vi "Athesim control.vi"() -> ()   [LabVIEW 2021]
uses:
  <vilib>/DAQmx/write.llb/DAQmx Write (Digital Bool 1Line 1Point).vi
  <vilib>/DAQmx/write.llb/DAQmx Write (Analog DBL 1Chan 1Samp).vi
  <vilib>/DAQmx/read.llb/DAQmx Read (Digital Bool 1Line 1Point).vi
  <vilib>/DAQmx/write.llb/DAQmx Write (Analog Wfm 1Chan NSamp).vi
  <vilib>/DAQmx/create/channels.llb/DAQmx Create Channel (DO-Digital Output).vi
  <vilib>/DAQmx/create/channels.llb/DAQmx Create Channel (DI-Digital Input).vi
  <vilib>/DAQmx/create/channels.llb/DAQmx Create Channel (AO-Voltage-Basic).vi
  <vilib>/DAQmx/miscellaneous.llb/DAQmx Fill In Error Info.vi
  <vilib>/Instr/_visa.llb/VISA Configure Serial Port (Instr).vi
  <vilib>/measure/NI_MABase.lvlib
panel:
  out "?":bool
  in  "Go live":bool
  in  "stop":bool=TRUE
  in  "Go SIM":bool
  in  "MG17Motor":refnum<k7>(container)
  in  "Tab Control":T1(tab)
  in  "Jog Z":bool
  in  "acquire 405":bool
  in  "405 Exp":dbl=150.0
  out "Images needed":dbl=216.0
  in  "5 phases":bool
  in  "Exposure time":dbl=100.0
  in  "interval /s":dbl
  in  "Timepoints":u32=8 min=1 max=1000 step=1
  in  "647":bool
  in  "561":bool
  in  "488":bool
  in  "405":bool
  in  "Steps /um":dbl
  in  "z-slices":dbl=1.0
  in  "acquire 640":bool
  in  "647 Exp":dbl=150.0
  in  "acquire 561":bool=TRUE
  in  "561 Exp":dbl=80.0
  in  "acquire 488":bool
  in  "488 Exp":dbl=40.0
  in  "Live mode":enum32{"Static", "Strobe", "Widefield", "SIM"}(radio)
  in  "Settle time":u32=60
  in  "Optosplit":T2(radio)=enum."rolling SIM"
  out "odd/even indicator":bool=TRUE
  out "Current voltage":dbl=0.95 format="%#_13g"
  in  "Boolean":bool
  in  "Radio Buttons":enum32{"V1", "V2", "V3"}(radio)
  in  "Debug":dbl[](array[numeric])=[0.95, 2.2, 3.45]
  in  "647 voltages":dbl[][](array[numeric])=[[0.95, 2.25, 3.5], [0.950655, 2.25185, 3.50055], [0.95131, 2.2537, 3.5011]]
  in  "561 voltages":dbl[][](array[numeric])=[[0.95, 2.2, 3.45], [0.9506, 2.2018, 3.451], [0.9512, 2.204, 3.452]]
  in  "488 voltages":dbl[][](array[numeric])=[[0.95, 2.25, 3.5], [0.951, 2.25185, 3.50055], [0.952, 2.2537, 3.5011]]
  in  "405 voltages":dbl[][](array[numeric])=[[1.0, 0.0, 0.0], [0.0, 0.0, 0.0], [0.0, 0.0, 4.0]]
  out "x+y":i32=5
  in  "647 voltages":dbl[][](array[numeric])=[[0.96, 2.2, 3.5], [0.97, 2.2035, 3.5085], [0.975, 2.2045, 3.5118]]
  in  "561 voltages":dbl[][](array[numeric])=[[0.85, 1.91, 3.2], [0.85065, 1.91064, 3.204], [0.85013, 1.91128, 3.208]]
  in  "488 voltages":dbl[][](array[numeric])=[[0.96, 2.2, 3.5], [0.97, 2.2045, 3.51], [0.975, 2.209, 3.52]]
  in  "405 voltages":dbl[][](array[numeric])=[[1.0, 0.0, 0.0], [0.0, 0.0, 0.0], [0.0, 0.0, 4.0]]
  in  "488 channel":refnum<visa-resource-name>="COM7"
  in  "488 power":dbl(slide)=5.627705627705628 min=0.0 max=100.0 step=0.05 scale=0.0..100.0
  in  "ASI stage channel":refnum<visa-resource-name>="COM3"
  in  "physical channels":tag="Dev1/ao0"
  in  "expose any":tag="Dev1/port0/line5"
  in  "647 Power":ext(slide)=31.05 scale=0.0..100.0
  in  "405 shutter":tag="Dev1/port0/line8"
  in  "561 shutter":tag="Dev1/port0/line0"
  in  "488 shutter":tag="Dev1/port0/line1"
  in  "Busy in":tag="Dev1/port0/line3"
  in  "Exposure out":tag="Dev1/port0/line2"
  in  "647 channel":refnum<visa-resource-name>="COM5"
  in  "561 power":dbl(slide)=31.16883116883117 min=0.0 max=100.0 step=0.05 scale=0.0..100.0
  in  "Tab Control 2":T3(tab)=enum."Page 5"
  out "Initialisation error":errorcluster
  out "stage error":errorcluster
  out "Camera/galvo error":errorcluster
  out "Laser error":errorcluster
  out "optosplit stage error":errorcluster
  out "resulting string":string="movrel z=0.000000 \r\n"
  out "resulting string 2":string="movrel z=-0.000000 \r\n"
  in  "short delay":dbl=5.0
  in  "long delay":dbl=55.0
  # "Acquire mode"
  # "o"
  # "o"
  # "o"
  # "o"
  # "o"
  # "o"
  # "o"
  # "o"
  # "o"
  # "o"
  # "o"
  # "o"
  # "-60"
  # "0"
  # "60"
  # "-60"
  # "0"
  # "60"
  # "-60"
  # "0"
  # "60"
  # "-60"
  # "0"
  # "60"
  # "0"
  # "2p/3"
  # "4p/3"
  # "o"
  # "o"
  # "o"
  # "o"
  # "o"
  # "o"
  # "o"
  # "o"
  # "o"
  # "o"
  # "o"
  # "o"
  # "-60"
  # "0"
  # "60"
  # "-60"
  # "0"
  # "60"
  # "-60"
  # "0"
  # "60"
  # "-60"
  # "0"
  # "60"
  # "0"
  # "3p/5"
  # "5p/5"
  # "7p/5"
  # "9p/5"
  # "Hardware lines"
  # "Laser control"
  # "Camera lines"
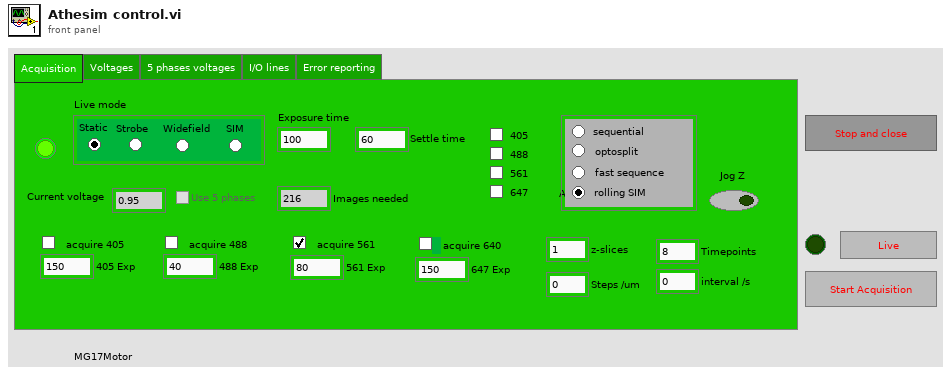
[diagram p1: front panel]
types:
  T1 = enum32{"Acquisition", "Voltages", "5 phases voltages", "I/O lines", "Error reporting"}
  T2 = enum32{"sequential", "optosplit", "fast sequence", "rolling SIM"}
  T3 = enum32{"Page 1", "Page 2", "Page 3", "Page 4", "Page 5"}
  T4 = enum8{"Enabled", "Disabled", "Disabled and Grayed Out"}
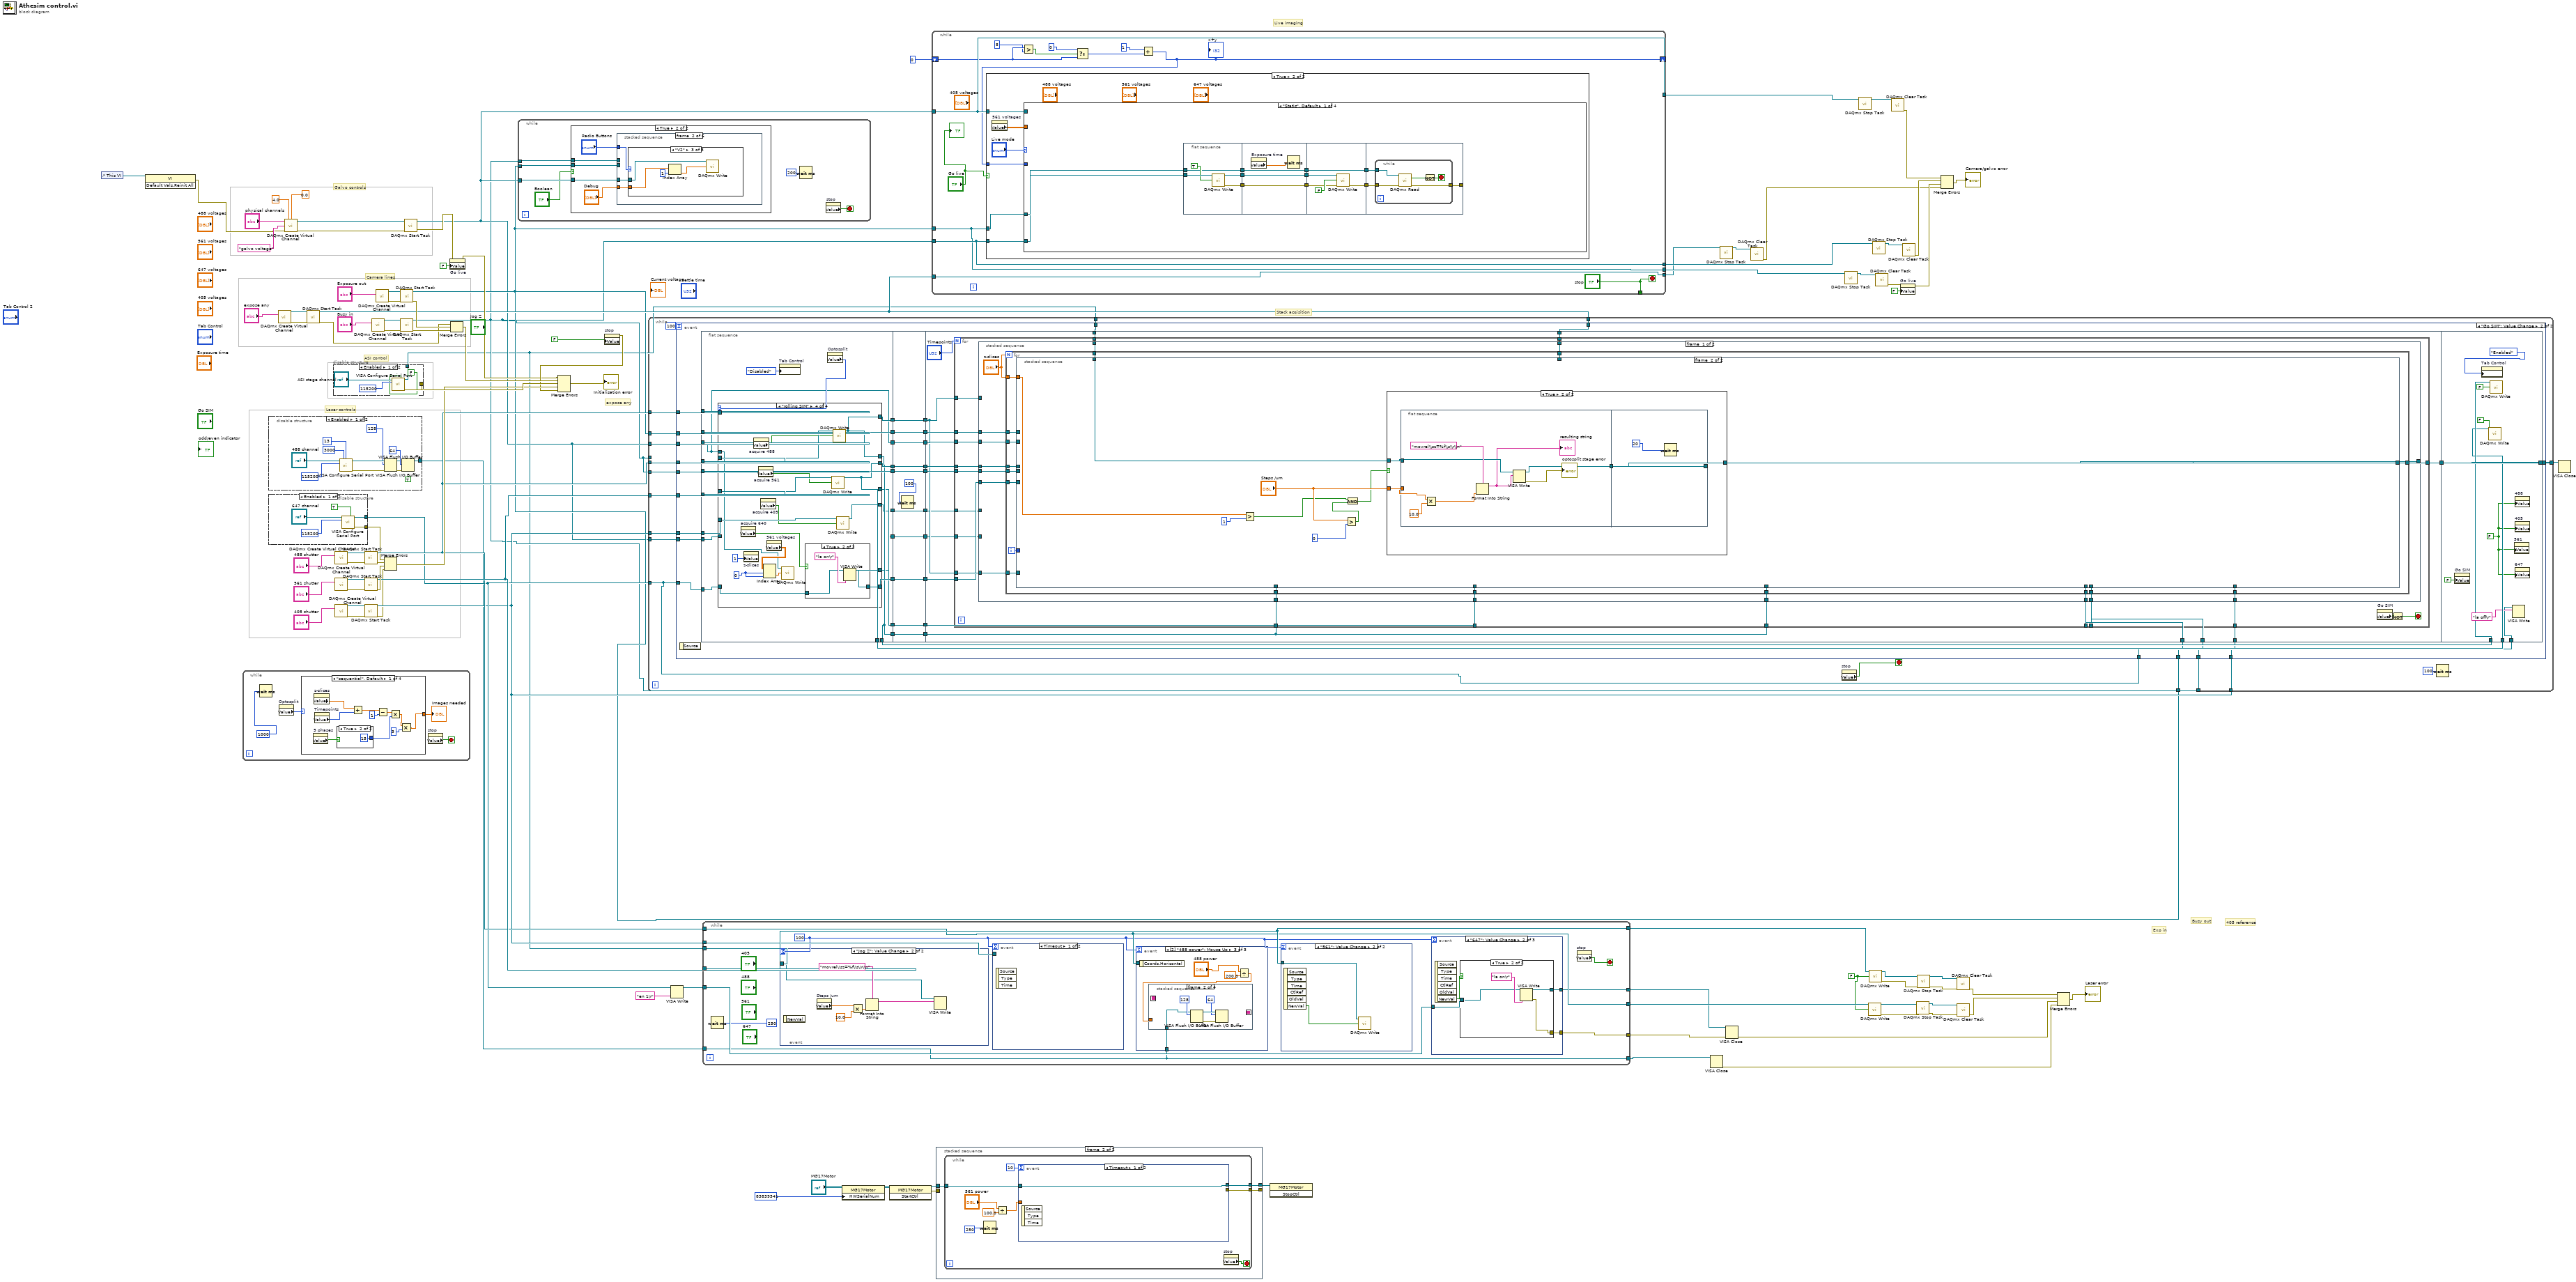
[diagram p0: block diagram]
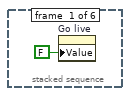
[diagram p4: hidden frame]
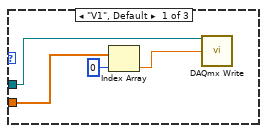
[diagram p5: hidden frame]
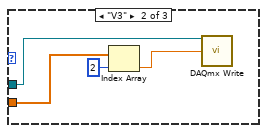
[diagram p6: hidden frame]
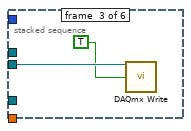
[diagram p7: hidden frame]
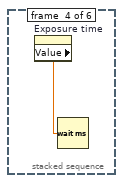
[diagram p8: hidden frame]
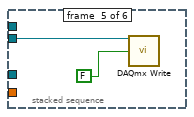
[diagram p9: hidden frame]
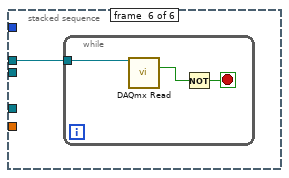
[diagram p10: hidden frame]
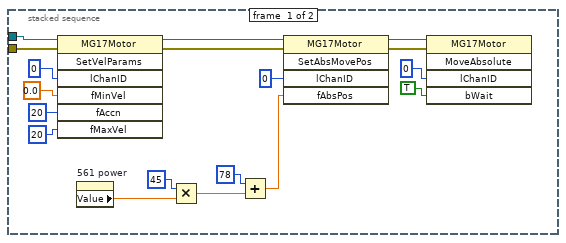
[diagram p11: hidden frame]
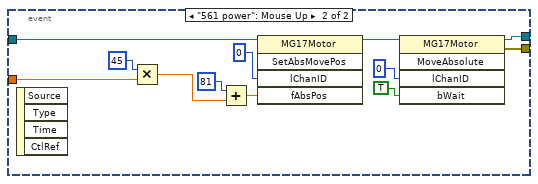
[diagram p12: hidden frame]
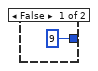
[diagram p14: hidden frame]
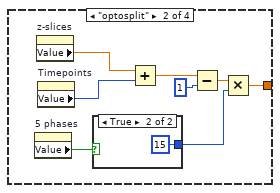
[diagram p15: hidden frame]
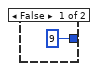
[diagram p16: hidden frame]
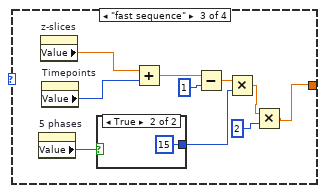
[diagram p17: hidden frame]
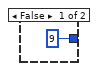
[diagram p18: hidden frame]
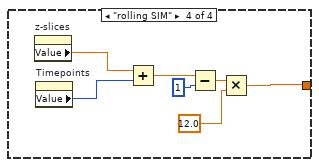
[diagram p19: hidden frame]
diagram:
  w63 = FALSE
  # "expose any"
  # "Busy out"
  # "Exp in"
  # "405 reference"
  # "Stack acqisition"
  # "Live imaging"
  # "Laser controls"
  # "ASI control"
  # "Camera lines"
  # "Galvo controls"
  n1 = control-ref of="This VI"() -> (w3:refnum<vi>)
  n2 = invoke class="VI" method="Default Vals.Reinit All"(reference=w3) -> (error out=w2:errorcluster)  [unwired: 2 in, 2 out]
  n3 = while {
    stop <- w99 stop-if-true
    n4 = Wait (ms)(milliseconds to wait=1000) -> ()  [unwired: 1 out]
    n5 = property on="Optosplit" class="RadioBtnsControl (strict)"() -> ("Value"=w98:T2)  [unwired: 2 in, 2 out]
    n6 = case shown="\"sequential\", Default" w98 {
      tunnel: [w101 w118 w123 w136] -> w100
      frame "sequential", Default {
        n7 = property on="5 phases" class="Bool (strict)"() -> ("Value"=w110:bool)  [unwired: 2 in, 2 out]
        n8 = property on="z-slices" class="DigNum (strict)"() -> ("Value"=w108:dbl)  [unwired: 2 in, 2 out]
        n9 = property on="Timepoints" class="DigNum (strict)"() -> ("Value"=w107:u32)  [unwired: 2 in, 2 out]
        n10 = case shown="True" w110 {
          tunnel: [9 15] -> w109
          frame False {
          }
          frame True {
          }
        }
        n11 = Add(x=w108, y=w107) -> (x+y=w105:dbl)
        n12 = Subtract(x=w105, y=1) -> (x-y=w104:dbl)
        n13 = Multiply(x=w104, y=w109) -> (x*y=w103:dbl)
        n14 = Multiply(x=w103, y=3) -> (x*y=w101:dbl)
      }
      frame "optosplit" {
        n15 = property on="5 phases" class="Bool (strict)"() -> ("Value"=w120:bool)  [unwired: 2 in, 2 out]
        n16 = property on="z-slices" class="DigNum (strict)"() -> ("Value"=w117:dbl)  [unwired: 2 in, 2 out]
        n17 = property on="Timepoints" class="DigNum (strict)"() -> ("Value"=w116:u32)  [unwired: 2 in, 2 out]
        n18 = case shown="True" w120 {
          tunnel: [9 15] -> w119
          frame False {
          }
          frame True {
          }
        }
        n19 = Add(x=w117, y=w116) -> (x+y=w114:dbl)
        n20 = Subtract(x=w114, y=1) -> (x-y=w113:dbl)
        n21 = Multiply(x=w113, y=w119) -> (x*y=w118:dbl)
      }
      frame "fast sequence" {
        n22 = property on="5 phases" class="Bool (strict)"() -> ("Value"=w132:bool)  [unwired: 2 in, 2 out]
        n23 = property on="z-slices" class="DigNum (strict)"() -> ("Value"=w130:dbl)  [unwired: 2 in, 2 out]
        n24 = property on="Timepoints" class="DigNum (strict)"() -> ("Value"=w129:u32)  [unwired: 2 in, 2 out]
        n25 = case shown="True" w132 {
          tunnel: [9 15] -> w131
          frame False {
          }
          frame True {
          }
        }
        n26 = Add(x=w130, y=w129) -> (x+y=w127:dbl)
        n27 = Subtract(x=w127, y=1) -> (x-y=w126:dbl)
        n28 = Multiply(x=w126, y=w131) -> (x*y=w125:dbl)
        n29 = Multiply(x=w125, y=2) -> (x*y=w123:dbl)
      }
      frame "rolling SIM" {
        n30 = property on="z-slices" class="DigNum (strict)"() -> ("Value"=w141:dbl)  [unwired: 2 in, 2 out]
        n31 = property on="Timepoints" class="DigNum (strict)"() -> ("Value"=w140:u32)  [unwired: 2 in, 2 out]
        n32 = Add(x=w141, y=w140) -> (x+y=w138:dbl)
        n33 = Subtract(x=w138, y=1) -> (x-y=w137:dbl)
        n34 = Multiply(x=w137, y=12.0) -> (x*y=w136:dbl)
      }
    }
    "Images needed" <- w100
    n35 = property on="stop" class="Bool (strict)"() -> ("Value"=w99:bool)  [unwired: 2 in, 2 out]
  }
  n36 = disable-structure shown="Enabled" {
    disable-tunnel: [w142 _] -> w7
    frame Enabled {
      (unwired) TRUE ("Enable Termination\nChar (T)")
      n37 = call-poly "VISA Configure Serial Port"("VISA resource name"="488 channel", "timeout (10sec)"=u32 3000, "termination char\n(0xA = '\\n' = LF)"=u8 13 ("termination char\n(0xA = '\\n' = LF)"), "baud rate (9600)"=u32 115200) -> ("VISA resource name out"=w152:refnum<visa-resource-name>, "error out"=w151:errorcluster)  [unwired: 5 in, 5 out]
      n38 = VISA Flush I/O Buffer(VISA resource name=w152, mask (16)=u16 128, error in (no error)=w151) -> (VISA resource name out=w148:refnum<visa-resource-name>, error out=w147:errorcluster)
      n39 = VISA Flush I/O Buffer(VISA resource name=w148, mask (16)=u16 64, error in (no error)=w147) -> (VISA resource name out=w142:refnum<visa-resource-name>)  [unwired: 1 out]
    }
    frame Disabled {
    }
  }
  n40 = disable-structure shown="Enabled" {
    disable-tunnel: [w154 _] -> w34
    disable-tunnel: [w153 _] -> w36
    frame Enabled {
      n41 = call-poly "VISA Configure Serial Port"("VISA resource name"="647 channel", "Enable Termination\nChar (T)"=TRUE ("Enable Termination\nChar (T)"), "baud rate (9600)"=u32 115200) -> ("VISA resource name out"=w154:refnum<visa-resource-name>, "error out"=w153:errorcluster)  [unwired: 11 in]
    }
    frame Disabled {
    }
  }
  n42 = call-poly <vilib>:"DAQmx Create Virtual Channel.vi"("lines"="expose any") -> ("task out"=w20:refnum<k21>, "error out"=w19:errorcluster)  [unwired: 13 in]
  n43 = call-poly <vilib>:"DAQmx Create Virtual Channel.vi"("maximum value"=4.0, "minimum value"=0.0, "physical channels"="physical channels", "name to assign"="galvo voltage", "error in"=w2) -> ("task out"=w13:refnum<k21>, "error out"=w12:errorcluster)  [unwired: 9 in]
  n44 = call <vilib>:"DAQmx Start Task.vi"("task/channels in"=w20, "error in"=w19) -> ("task out"=w17:refnum<k21>, "error out"=w18:errorcluster)  [unwired: 12 in]
  n45 = disable-structure shown="Enabled" {
    disable-tunnel: [w160 _] -> w80
    disable-tunnel: [w159 _] -> w1
    frame Enabled {
      n46 = call-poly "VISA Configure Serial Port"("VISA resource name"="ASI stage channel", "Enable Termination\nChar (T)"=FALSE, "baud rate (9600)"=u32 115200) -> ("VISA resource name out"=w159:refnum<visa-resource-name>, "error out"=w160:errorcluster)  [unwired: 11 in]
    }
    frame Disabled {
    }
  }
  n47 = call-poly <vilib>:"DAQmx Create Virtual Channel.vi"("lines"="488 shutter") -> ("task out"=w91:refnum<k21>, "error out"=w92:errorcluster)  [unwired: 13 in]
  n48 = call-poly <vilib>:"DAQmx Create Virtual Channel.vi"("lines"="561 shutter") -> ("task out"=w89:refnum<k21>, "error out"=w90:errorcluster)  [unwired: 13 in]
  n49 = call-poly <vilib>:"DAQmx Create Virtual Channel.vi"("lines"="405 shutter") -> ("task out"=w46:refnum<k21>, "error out"=w47:errorcluster)  [unwired: 13 in]
  n50 = call <vilib>:"DAQmx Start Task.vi"("task/channels in"=w91, "error in"=w92) -> ("task out"=w75:refnum<k21>, "error out"=w84:errorcluster)  [unwired: 12 in]
  n51 = call <vilib>:"DAQmx Start Task.vi"("task/channels in"=w89, "error in"=w90) -> ("task out"=w76:refnum<k21>, "error out"=w83:errorcluster)  [unwired: 12 in]
  n52 = call <vilib>:"DAQmx Start Task.vi"("task/channels in"=w46, "error in"=w47) -> ("task out"=w32:refnum<k21>, "error out"=w8:errorcluster)  [unwired: 12 in]
  n53 = call-poly <vilib>:"DAQmx Create Virtual Channel.vi"("lines"="Busy in") -> ("task out"=w93:refnum<k21>, "error out"=w94:errorcluster)  [unwired: 13 in]
  n54 = call-poly <vilib>:"DAQmx Create Virtual Channel.vi"("lines"="Exposure out") -> ("task out"=w96:refnum<k21>, "error out"=w95:errorcluster)  [unwired: 13 in]
  n55 = Merge Errors(w36, w84, w83, w8) -> (w78:errorcluster)
  n56 = call <vilib>:"DAQmx Start Task.vi"("task/channels in"=w96, "error in"=w95) -> ("task out"=w10:refnum<k21>, "error out"=w82:errorcluster)  [unwired: 12 in]
  n57 = call <vilib>:"DAQmx Start Task.vi"("task/channels in"=w93, "error in"=w94) -> ("task out"=w4:refnum<k21>, "error out"=w81:errorcluster)  [unwired: 12 in]
  n58 = call <vilib>:"DAQmx Start Task.vi"("task/channels in"=w13, "error in"=w12) -> ("task out"=w9:refnum<k21>, "error out"=w30:errorcluster)  [unwired: 12 in]
  n59 = property on="Go live" class="Bool (strict)"(error in=w30, "Value"=FALSE) -> (error out=w29:errorcluster)  [unwired: 1 in, 1 out]
  n60 = Merge Errors(w18, w82, w81) -> (w79:errorcluster)
  n61 = while {
    tunnel: w10 -> [w167]
    tunnel: w4 -> [w166]
    tunnel: w9 -> [w165]
    stop <- w168 stop-if-true
    n62 = case shown="True" "Boolean" {
      tunnel: w167 -> [_ w173]
      tunnel: w166 -> [_ w172]
      tunnel: w165 -> [_ w171]
      frame False {
      }
      frame True {
        n63 = stacked-sequence {
          tunnel: w173 -> [_ _ w191 _ w193 _]
          tunnel: w172 -> [_ _ _ _ _ w195]
          tunnel: "Radio Buttons" -> [_ w177 _ _ _ _]
          tunnel: "Debug" -> [_ w176 _ _ _ _]
          tunnel: w171 -> [_ w175 _ _ _ _]
          frame #0 {
            n64 = property on="Go live" class="Bool (strict)"("Value"=FALSE ("Go live")) -> ()  [unwired: 2 in, 2 out]
          }
          frame #1 {
            n65 = case shown="\"V2\"" w177 {
              tunnel: w176 -> [w180 w184 w188]
              tunnel: w175 -> [w181 w185 w189]
              frame "V1", Default {
                n66 = Index Array(array=w180, index=0) -> (element=w179:dbl)
                n67 = call-poly <vilib>:"DAQmx Write.vi"("task/channels in"=w181, "data"=w179) -> ()  [unwired: 11 in, 3 out]
              }
              frame "V3" {
                n68 = Index Array(array=w184, index=2) -> (element=w183:dbl)
                n69 = call-poly <vilib>:"DAQmx Write.vi"("task/channels in"=w185, "data"=w183) -> ()  [unwired: 11 in, 3 out]
              }
              frame "V2" {
                n70 = Index Array(array=w188, index=1) -> (element=w187:dbl)
                n71 = call-poly <vilib>:"DAQmx Write.vi"("task/channels in"=w189, "data"=w187) -> ()  [unwired: 11 in, 3 out]
              }
            }
          }
          frame #2 {
            n72 = call-poly <vilib>:"DAQmx Write.vi"("task/channels in"=w191, "data"=TRUE) -> ()  [unwired: 11 in, 3 out]
          }
          frame #3 {
            n73 = property on="Exposure time" class="DigNum (strict)"() -> ("Value"=w192:dbl)  [unwired: 2 in, 2 out]
            n74 = Wait (ms)(milliseconds to wait=w192) -> ()  [unwired: 1 out]
          }
          frame #4 {
            n75 = call-poly <vilib>:"DAQmx Write.vi"("task/channels in"=w193, "data"=FALSE) -> ()  [unwired: 11 in, 3 out]
          }
          frame #5 {
            n76 = while {
              tunnel: w195 -> [w196]
              stop <- w198 stop-if-true
              n77 = call-poly <vilib>:"DAQmx Read.vi"("task/channels in"=w196) -> ("data"=w197:bool)  [unwired: 12 in, 2 out]
              n78 = Not(x=w197) -> (.not. x?=w198:bool)
            }
          }
        }
      }
    }
    n79 = Wait (ms)(milliseconds to wait=u32 200) -> ()  [unwired: 1 out]
    n80 = property on="stop" class="Bool (strict)"() -> ("Value"=w168:bool)  [unwired: 2 in, 2 out]
  }
  n81 = property on="stop" class="Bool (strict)"("Value"=FALSE) -> (error out=w49:errorcluster)  [unwired: 2 in, 1 out]
  n82 = Merge Errors(w29, w79, w80, w78, w49) -> (→"Initialisation error":errorcluster)
  n83 = while {
    tunnel: w10 -> [w215]
    tunnel: w4 -> [w214]
    tunnel: w9 -> [w213]
    tunnel: w75 -> [w212]
    tunnel: w76 -> [w211]
    tunnel: w75 -> [w210]
    tunnel: w1 -> [w208]
    tunnel: [w207] -> w51
    tunnel: w4 -> [_]
    tunnel: w34 -> [w205]
    tunnel: w32 -> [w206]
    tunnel: w32 -> [w204]
    tunnel: w10 -> [w203]
    tunnel: w4 -> [w202]
    tunnel: w9 -> [w201]
    tunnel: w17 -> [w200]
    stop <- w209 stop-if-true
    n84 = event shown="[1] \"Go SIM\": Value Change" {
      selector: _ -> [_ _]
      dyn-events: _ -> [_ _]
      timeout: 100 -> [_ _]
      tunnel: w215 -> [_ w256]
      tunnel: w214 -> [_ w255]
      tunnel: w213 -> [_ w254]
      tunnel: w212 -> [_ w253]
      tunnel: w211 -> [_ w252]
      tunnel: w210 -> [_ w251]
      tunnel: w208 -> [w217 w250]
      tunnel: [w217 w249] -> w207
      tunnel: w205 -> [_ w245]
      tunnel: w206 -> [_ w244]
      tunnel: w205 -> [_ w243]
      tunnel: w204 -> [_ w242]
      tunnel: w203 -> [_ w241]
      tunnel: w202 -> [_ w240]
      tunnel: w201 -> [_ w239]
      tunnel: w200 -> [_ w218]
      event Timeout {
        n85 = event-data() -> ()  [unwired: 1 in, 3 out]
      }
      event "Go SIM": Value Change {
        n86 = event-data() -> ()  [unwired: 1 in, 1 out]
        n87 = flat-sequence {
          tunnel: [w274] -> w238
          tunnel: w256 -> [w274]
          tunnel: [w273] -> w236
          tunnel: w255 -> [w273]
          tunnel: [w258] -> w234
          tunnel: w254 -> [w258]
          tunnel: w253 -> [w271]
          tunnel: w252 -> [w270]
          tunnel: w251 -> [w269]
          tunnel: [w268] -> w232
          tunnel: [w267] -> w230
          tunnel: [w263] -> w246
          tunnel: [w262] -> w247
          tunnel: w245 -> [w266]
          tunnel: w244 -> [w265]
          tunnel: [w264] -> w228
          tunnel: [w263] -> w226
          tunnel: [w262] -> w224
          tunnel: w239 -> [w261]
          tunnel: [w260] -> w221
          tunnel: [w259] -> w219
          tunnel: w238 -> [w364]
          tunnel: [w364] -> w237
          tunnel: w236 -> [w363]
          tunnel: [w363] -> w235
          tunnel: w234 -> [w362]
          tunnel: [w362] -> w233
          tunnel: w232 -> [w361]
          tunnel: [w361] -> w231
          tunnel: w230 -> [w360]
          tunnel: [w360] -> w229
          tunnel: w228 -> [w359]
          tunnel: [w359] -> w227
          tunnel: w226 -> [w358]
          tunnel: [w358] -> w225
          tunnel: w224 -> [w357]
          tunnel: [w357] -> w223
          tunnel: [w355] -> w222
          tunnel: w221 -> [w355]
          tunnel: [w354] -> w220
          tunnel: w219 -> [w354]
          tunnel: w237 -> [w381]
          tunnel: w235 -> [w380]
          tunnel: w233 -> [w379]
          tunnel: w231 -> [w378]
          tunnel: w229 -> [w369]
          tunnel: w250 -> [w377]
          tunnel: [w376] -> w248
          tunnel: w227 -> [w375]
          tunnel: w225 -> [w373]
          tunnel: w223 -> [w374]
          tunnel: w242 -> [w372]
          tunnel: w241 -> [w371]
          tunnel: w240 -> [w370]
          tunnel: w222 -> [w368]
          tunnel: w220 -> [w367]
          tunnel: w218 -> [w366]
          tunnel: [w1177] -> w249
          tunnel: w248 -> [w1177]
          tunnel: w247 -> [w1173]
          tunnel: w246 -> [w1174]
          tunnel: w243 -> [w1171]
          frame #0 {
            n88 = property on="Tab Control" class="TabCtl (strict)"("DisabledEnum"=T4."Disabled" ("Disabled")) -> ()  [unwired: 2 in, 2 out]
            n89 = property on="Optosplit" class="RadioBtnsControl (strict)"() -> ("Value"=w272:T2)  [unwired: 2 in, 2 out]
            n90 = case shown="\"rolling SIM\"" w272 {
              tunnel: w271 -> [_ _ _ _]
              tunnel: w270 -> [w285 w307 w326 w345]
              tunnel: w269 -> [w286 w308 w328 w347]
              tunnel: [w284 w306 w325 w344] -> w268
              tunnel: [w283 w305 w327 w346] -> w267
              tunnel: [w284 w306 w325 w344] -> w262
              tunnel: [w283 w305 w327 w346] -> w263
              tunnel: w266 -> [w278 w300 w323 w343]
              tunnel: w265 -> [w281 w303 w321 w342]
              tunnel: [w275 w297 w319 w340] -> w264
              tunnel: [w279 w301 w320 w341] -> w260
              tunnel: w261 -> [w276 w299 _ _]
              tunnel: [w275 w297 w319 w340] -> w259
              tunnel: w258 -> [_ _ _ w331]
              frame "sequential", Default {
                n91 = property on="odd/even indicator" class="Bool (strict)"() -> ("Value"=w277:bool)  [unwired: 2 in, 2 out]
                n92 = case shown="True" w277 {
                  tunnel: w276 -> [w292 w296]
                  frame False {
                    w290 = 2
                    n93 = property on="647 voltages" class="Arr (strict)"() -> ("Value"=w291:dbl[][])  [unwired: 2 in, 2 out]
                    n94 = Index Array(array=w291, index (row)=w290, index (col)=w290) -> (element=w289:dbl)
                    n95 = call-poly <vilib>:"DAQmx Write.vi"("task/channels in"=w292, "data"=w289) -> ()  [unwired: 11 in, 3 out]
                  }
                  frame True {
                    w294 = 0
                    n96 = property on="561 voltages" class="Arr (strict)"() -> ("Value"=w295:dbl[][])  [unwired: 2 in, 2 out]
                    n97 = Index Array(array=w295, index (row)=w294, index (col)=w294) -> (element=w293:dbl)
                    n98 = call-poly <vilib>:"DAQmx Write.vi"("task/channels in"=w296, "data"=w293) -> ()  [unwired: 11 in, 3 out]
                  }
                }
                n99 = call-poly <vilib>:"DAQmx Write.vi"("task/channels in"=w281, "data"=FALSE) -> ("task out"=w279:refnum<k21>)  [unwired: 11 in, 2 out]
                n100 = call-poly <vilib>:"DAQmx Write.vi"("task/channels in"=w285, "data"=FALSE) -> ("task out"=w284:refnum<k21>)  [unwired: 11 in, 2 out]
                n101 = call-poly <vilib>:"DAQmx Write.vi"("task/channels in"=w286, "data"=FALSE) -> ("task out"=w283:refnum<k21>)  [unwired: 11 in, 2 out]
                n102 = VISA Write(VISA resource name=w278, write buffer="la off\r" ("format string")) -> (VISA resource name out=w275:refnum<visa-resource-name>)  [unwired: 1 in, 2 out]
              }
              frame "fast sequence" {
                n103 = property on="odd/even indicator" class="Bool (strict)"() -> ("Value"=w298:bool)  [unwired: 2 in, 2 out]
                n104 = case shown="True" w298 {
                  tunnel: w299 -> [w314 w318]
                  frame False {
                    w312 = 2
                    n105 = property on="647 voltages" class="Arr (strict)"() -> ("Value"=w313:dbl[][])  [unwired: 2 in, 2 out]
                    n106 = Index Array(array=w313, index (row)=w312, index (col)=w312) -> (element=w311:dbl)
                    n107 = call-poly <vilib>:"DAQmx Write.vi"("task/channels in"=w314, "data"=w311) -> ()  [unwired: 11 in, 3 out]
                  }
                  frame True {
                    w316 = 0
                    n108 = property on="647 voltages" class="Arr (strict)"() -> ("Value"=w317:dbl[][])  [unwired: 2 in, 2 out]
                    n109 = Index Array(array=w317, index (row)=w316, index (col)=w316) -> (element=w315:dbl)
                    n110 = call-poly <vilib>:"DAQmx Write.vi"("task/channels in"=w318, "data"=w315) -> ()  [unwired: 11 in, 3 out]
                  }
                }
                n111 = call-poly <vilib>:"DAQmx Write.vi"("task/channels in"=w303, "data"=FALSE) -> ("task out"=w301:refnum<k21>)  [unwired: 11 in, 2 out]
                n112 = call-poly <vilib>:"DAQmx Write.vi"("task/channels in"=w307, "data"=FALSE) -> ("task out"=w306:refnum<k21>)  [unwired: 11 in, 2 out]
                n113 = call-poly <vilib>:"DAQmx Write.vi"("task/channels in"=w308, "data"=FALSE) -> ("task out"=w305:refnum<k21>)  [unwired: 11 in, 2 out]
                n114 = VISA Write(VISA resource name=w300, write buffer="la off\r" ("format string")) -> (VISA resource name out=w297:refnum<visa-resource-name>)  [unwired: 1 in, 2 out]
              }
              frame "optosplit" {
                n115 = call-poly <vilib>:"DAQmx Write.vi"("task/channels in"=w326, "data"=TRUE) -> ("task out"=w325:refnum<k21>)  [unwired: 11 in, 2 out]
                n116 = call-poly <vilib>:"DAQmx Write.vi"("task/channels in"=w328, "data"=TRUE) -> ("task out"=w327:refnum<k21>)  [unwired: 11 in, 2 out]
                n117 = call-poly <vilib>:"DAQmx Write.vi"("task/channels in"=w321, "data"=TRUE) -> ("task out"=w320:refnum<k21>)  [unwired: 11 in, 2 out]
                n118 = VISA Write(VISA resource name=w323, write buffer="la on\r" ("format string")) -> (VISA resource name out=w319:refnum<visa-resource-name>)  [unwired: 1 in, 2 out]
              }
              frame "rolling SIM" {
                w336 = 0
                n119 = property on="acquire 640" class="Bool (strict)"() -> ("Value"=w332:bool)  [unwired: 2 in, 2 out]
                n120 = property on="z-slices" class="DigNum (strict)"("Value"=1) -> ()  [unwired: 2 in, 2 out]
                n121 = property on="acquire 488" class="Bool (strict)"() -> ("Value"=w335:bool)  [unwired: 2 in, 2 out]
                n122 = property on="acquire 561" class="Bool (strict)"() -> ("Value"=w334:bool)  [unwired: 2 in, 2 out]
                n123 = property on="acquire 405" class="Bool (strict)"() -> ("Value"=w333:bool)  [unwired: 2 in, 2 out]
                n124 = property on="561 voltages" class="Arr (strict)"() -> ("Value"=w337:dbl[][])  [unwired: 2 in, 2 out]
                n125 = Index Array(array=w337, index (row)=w336, index (col)=w336) -> (element=w338:dbl)
                n126 = call-poly <vilib>:"DAQmx Write.vi"("task/channels in"=w331, "data"=w338) -> ()  [unwired: 11 in, 3 out]
                n127 = case shown="True" w332 {
                  tunnel: w343 -> [w349 w352]
                  tunnel: [w348 w351] -> w340
                  frame False {
                    n128 = VISA Write(VISA resource name=w349, write buffer="la off\r" ("format string")) -> (VISA resource name out=w348:refnum<visa-resource-name>)  [unwired: 1 in, 2 out]
                  }
                  frame True {
                    n129 = VISA Write(VISA resource name=w352, write buffer="la on\r" ("format string")) -> (VISA resource name out=w351:refnum<visa-resource-name>)  [unwired: 1 in, 2 out]
                  }
                }
                n130 = call-poly <vilib>:"DAQmx Write.vi"("task/channels in"=w345, "data"=w334) -> ("task out"=w344:refnum<k21>)  [unwired: 11 in, 2 out]
                n131 = call-poly <vilib>:"DAQmx Write.vi"("task/channels in"=w347, "data"=w335) -> ("task out"=w346:refnum<k21>)  [unwired: 11 in, 2 out]
                n132 = call-poly <vilib>:"DAQmx Write.vi"("task/channels in"=w342, "data"=w333) -> ("task out"=w341:refnum<k21>)  [unwired: 11 in, 2 out]
              }
            }
          }
          frame #1 {
            n133 = Wait (ms)(milliseconds to wait=100) -> ()  [unwired: 1 out]
          }
          frame #2 {
            n134 = for {
              N: "Timepoints" -> [_]
              tunnel: w381 -> [w401]
              tunnel: w380 -> [w400]
              tunnel: w379 -> [w399]
              tunnel: w378 -> [w398]
              tunnel: w369 -> [w397]
              tunnel: w377 -> [w396]
              tunnel: [w395] -> w376
              tunnel: w375 -> [w394]
              tunnel: w374 -> [w393]
              tunnel: w373 -> [w392]
              tunnel: w373 -> [w391]
              tunnel: w372 -> [w390]
              tunnel: w371 -> [w389]
              tunnel: w370 -> [w388]
              tunnel: w369 -> [w387]
              tunnel: w368 -> [w386]
              tunnel: w367 -> [w385]
              tunnel: w366 -> [w384]
              stop <- w382 stop-if-true
              n135 = stacked-sequence {
                tunnel: w401 -> [w417 _]
                tunnel: w400 -> [w416 _]
                tunnel: w399 -> [w415 _]
                tunnel: w398 -> [w414 w1081]
                tunnel: w397 -> [w413 _]
                tunnel: w396 -> [w412 w1083]
                tunnel: [w411 _] -> w395
                tunnel: w394 -> [w410 _]
                tunnel: w393 -> [w409 _]
                tunnel: w392 -> [w408 _]
                tunnel: w391 -> [w407 _]
                tunnel: w390 -> [w406 _]
                tunnel: w389 -> [w405 _]
                tunnel: w388 -> [w404 _]
                tunnel: w387 -> [_ w1082]
                tunnel: w386 -> [_ w1080]
                tunnel: w385 -> [_ w1079]
                tunnel: w384 -> [w402 _]
                frame #0 {
                  n136 = for {
                    N: "z-slices" -> [_]
                    tunnel: w417 -> [w434]
                    tunnel: w416 -> [w433]
                    tunnel: w415 -> [w432]
                    tunnel: w414 -> [w431]
                    tunnel: w413 -> [w430]
                    tunnel: w412 -> [w429]
                    tunnel: [w428] -> w411
                    tunnel: w410 -> [w427]
                    tunnel: w409 -> [w426]
                    tunnel: w408 -> [w425]
                    tunnel: w407 -> [w424]
                    tunnel: w406 -> [w423]
                    tunnel: w405 -> [w422]
                    tunnel: w404 -> [w421]
                    tunnel: "z-slices" -> [w419]
                    tunnel: w402 -> [w418]
                    i -> [w420]
                    n137 = stacked-sequence {
                      tunnel: w434 -> [w449 _]
                      tunnel: w433 -> [w448 _]
                      tunnel: w432 -> [w447 _]
                      tunnel: w431 -> [w446 _]
                      tunnel: w430 -> [w445 _]
                      tunnel: w429 -> [_ w1051]
                      tunnel: [_ w1050] -> w428
                      tunnel: w427 -> [w443 _]
                      tunnel: w426 -> [w442 _]
                      tunnel: w425 -> [w441 _]
                      tunnel: w424 -> [w440 _]
                      tunnel: w423 -> [w439 _]
                      tunnel: w422 -> [w438 _]
                      tunnel: w421 -> [w437 _]
                      tunnel: w420 -> [w436 _]
                      tunnel: w419 -> [_ w1046]
                      tunnel: w418 -> [w435 _]
                      frame #0 {
                        n138 = case shown="\"rolling SIM\"" "Optosplit" {
                          tunnel: w449 -> [w472 w795 w924 w1021]
                          tunnel: w448 -> [w471 w794 w923 w1020]
                          tunnel: w447 -> [w454 w790 w922 w1014]
                          tunnel: w446 -> [w461 _ _ _]
                          tunnel: w445 -> [w460 _ _ _]
                          tunnel: "5 phases" -> [_ _ w921 _]
                          tunnel: w443 -> [w459 w789 _ _]
                          tunnel: w442 -> [w458 w788 _ _]
                          tunnel: w441 -> [w457 _ _ _]
                          tunnel: w440 -> [_ w783 _ _]
                          tunnel: w439 -> [w456 w782 _ _]
                          tunnel: w438 -> [w453 _ _ _]
                          tunnel: w437 -> [w452 _ _ _]
                          tunnel: w436 -> [_ _ _ _]
                          tunnel: w435 -> [w451 w781 w920 w1015]
                          frame "sequential", Default {
                            # "Without optosplit"
                            n139 = case shown="True" "acquire 640" {
                              tunnel: w472 -> [w700 w710]
                              tunnel: w471 -> [w698 w709]
                              tunnel: w454 -> [w699 w703]
                              tunnel: [w700 w707] -> w467
                              tunnel: [w699 w708] -> w468
                              tunnel: [w698 w706] -> w469
                              tunnel: w459 -> [_ w702]
                              tunnel: w451 -> [_ w701]
                              frame False {
                              }
                              frame True {
                                n140 = property on="647 voltages" class="Arr (strict)"() -> ("Value"=w704:dbl[][])  [unwired: 2 in, 2 out]
                                n141 = stacked-sequence {
                                seq-local: [_ w724 _ _] -> [_ _ w744 _]
                                seq-local: [_ w723 _ _] -> [_ _ w743 _]
                                seq-local: [_ w722 _ _] -> [_ _ w742 _]
                                seq-local: [_ w721 _ _] -> [_ _ w738 _]
                                seq-local: [_ w720 _ _] -> [_ _ w737 _]
                                tunnel: w710 -> [_ w724 _ _]
                                tunnel: w703 -> [_ w723 _ _]
                                tunnel: w709 -> [_ w722 _ _]
                                tunnel: w704 -> [_ w721 _ _]
                                tunnel: "647 Exp" -> [_ w720 _ _]
                                tunnel: [_ _ w741 _] -> w708
                                tunnel: [_ _ w740 _] -> w707
                                tunnel: [_ _ w739 _] -> w706
                                tunnel: w704 -> [_ w719 _ _]
                                tunnel: w703 -> [_ w718 _ _]
                                tunnel: w702 -> [w711 _ _ w778]
                                tunnel: w701 -> [_ _ w735 _]
                                frame #0 {
                                n142 = stacked-sequence {
                                tunnel: w711 -> [w712 _]
                                frame #0 {
                                n143 = VISA Write(VISA resource name=w712, write buffer="la on\r" ("format string")) -> ()  [unwired: 1 in, 3 out]
                                }
                                frame #1 {
                                n144 = Wait (ms)(milliseconds to wait=100) -> ()  [unwired: 1 out]
                                }
                                }
                                }
                                frame #1 {
                                n145 = property on="odd/even indicator" class="Bool (strict)"() -> ("Value"=w715:bool)  [unwired: 2 in, 2 out]
                                n146 = case shown="False" w715 {
                                tunnel: [2 0] -> w717
                                tunnel: [2 0] -> w716
                                frame False {
                                }
                                frame True {
                                }
                                }
                                n147 = flat-sequence {
                                tunnel: [w732] -> _
                                tunnel: w719 -> [w734]
                                tunnel: w718 -> [w732]
                                tunnel: [w733] -> _
                                tunnel: w717 -> [w730]
                                tunnel: w716 -> [w729]
                                frame #0 {
                                n148 = Index Array(array=w734, index (row)=w730, index (col)=w729) -> (element=w731:dbl)
                                n149 = call-poly <vilib>:"DAQmx Write.vi"("task/channels in"=w732, "data"=w731) -> ("task out"=w733:refnum<k21>)  [unwired: 11 in, 2 out]
                                }
                                }
                                }
                                frame #2 {
                                n150 = for {
                                N: 9 -> [_]
                                tunnel: w738 -> [w756]
                                tunnel: w744 -> [w753]
                                tunnel: w743 -> [w754]
                                tunnel: w742 -> [w752]
                                tunnel: w737 -> [w755]
                                tunnel: [w754] -> w741
                                tunnel: [w753] -> w740
                                tunnel: [w752] -> w739
                                tunnel: w735 -> [w745]
                                i -> [w748]
                                n151 = property on="odd/even indicator" class="Bool (strict)"() -> ("Value"=w746:bool)  [unwired: 2 in, 2 out]
                                n152 = case shown="True" w746 {
                                tunnel: [i32[] [1, 0, 2, 1, 0, 2, 1, 0, 0, 0, 1, 2, 3, 4, 0] i32[] [1, 2, 0, 1, 2, 0, 1, 2, 2, 0, 1, 2, 3, 4, 0]] -> w751
                                tunnel: [i32[] [2, 2, 1, 1, 1, 0, 0, 0, 0, 2, 2, 2, 2, 2, 0] i32[] [0, 0, 1, 1, 1, 2, 2, 2, 2, 2, 2, 2, 2, 2, 0]] -> w750
                                frame False {
                                }
                                frame True {
                                }
                                }
                                n153 = Index Array(array=w751, index=w748) -> (element=w749:i32)
                                n154 = flat-sequence {
                                tunnel: w756 -> [w765]
                                tunnel: w755 -> [w769]
                                tunnel: w754 -> [w768]
                                tunnel: w753 -> [w767]
                                tunnel: w752 -> [w766]
                                tunnel: w747 -> [w763]
                                tunnel: w749 -> [w762]
                                tunnel: w745 -> [w761]
                                frame #0 {
                                n155 = Index Array(array=w765, index (row)=w762, index (col)=w763) -> (element=w764:dbl)
                                n156 = call "take image.vi"("Voltage"=w764, "Exposure time"=w769, "expose any"=w761, "Busy out"=w766, "Exp In"=w767, "Galvo"=w768) -> ()  [unwired: 6 in]
                                }
                                frame #1 {
                                n157 = property on="Settle time" class="DigNum (strict)"() -> ("Value"=w770:u32)  [unwired: 2 in, 2 out]
                                n158 = Wait (ms)(milliseconds to wait=w770) -> ()  [unwired: 1 out]
                                }
                                }
                                n159 = Index Array(array=w750, index=w748) -> (element=w747:i32)
                                }
                                }
                                frame #3 {
                                n160 = property on="acquire 488" class="Bool (strict)"() -> ("Value"=w774:bool)  [unwired: 2 in, 2 out]
                                n161 = property on="acquire 405" class="Bool (strict)"() -> ("Value"=w773:bool)  [unwired: 2 in, 2 out]
                                n162 = property on="acquire 561" class="Bool (strict)"() -> ("Value"=w775:bool)  [unwired: 2 in, 2 out]
                                n163 = property on="odd/even indicator" class="Bool (strict)"() -> ("Value"=w776:bool)  [unwired: 2 in, 2 out]
                                n164 = Or(x=w775, y=w774) -> (x .or. y?=w772:bool)
                                n165 = Not(x=w776) -> (.not. x?=w777:bool)
                                n166 = Or(x=w772, y=w773) -> (x .or. y?=w771:bool)
                                n167 = case shown="True" w771 {
                                tunnel: w778 -> [_ w779]
                                frame False {
                                }
                                frame True {
                                n168 = VISA Write(VISA resource name=w779, write buffer="la off\r" ("format string")) -> ()  [unwired: 1 in, 3 out]
                                }
                                }
                                n169 = property on="odd/even indicator" class="Bool (strict)"("Value"=w777) -> ()  [unwired: 2 in, 2 out]
                                }
                                }
                              }
                            }
                            n170 = case shown="True" "acquire 561" {
                              tunnel: w469 -> [w617 w628]
                              tunnel: w468 -> [w618 w629]
                              tunnel: [w616 w626] -> w465
                              tunnel: [w618 w627] -> w464
                              tunnel: [w617 w625] -> w463
                              tunnel: w467 -> [w616 w624]
                              tunnel: w461 -> [_ _]
                              tunnel: w454 -> [_ w621]
                              tunnel: w458 -> [_ w620]
                              tunnel: w451 -> [_ w619]
                              frame False {
                              }
                              frame True {
                                n171 = property on="561 voltages" class="Arr (strict)"() -> ("Value"=w622:dbl[][])  [unwired: 2 in, 2 out]
                                n172 = stacked-sequence {
                                seq-local: [_ w639 _ _] -> [_ _ w661 _]
                                seq-local: [_ w638 _ _] -> [_ _ w660 _]
                                seq-local: [_ w637 _ _] -> [_ _ w656 _]
                                seq-local: [_ w636 _ _] -> [_ _ w654 _]
                                seq-local: [_ w635 _ _] -> [_ _ w653 _]
                                tunnel: w629 -> [_ w639 _ _]
                                tunnel: w628 -> [_ w638 _ _]
                                tunnel: w624 -> [_ w637 _ _]
                                tunnel: w622 -> [_ w636 _ _]
                                tunnel: "561 Exp" -> [_ w635 _ _]
                                tunnel: [_ _ w659 _] -> w627
                                tunnel: [_ _ w658 _] -> w626
                                tunnel: [_ _ w657 _] -> w625
                                tunnel: w622 -> [_ w633 _ _]
                                tunnel: w621 -> [_ w632 _ _]
                                tunnel: w620 -> [w631 _ _ w695]
                                tunnel: w619 -> [_ _ w652 _]
                                frame #0 {
                                n173 = call-poly <vilib>:"DAQmx Write.vi"("task/channels in"=w631, "data"=TRUE) -> ()  [unwired: 11 in, 3 out]
                                }
                                frame #1 {
                                n174 = flat-sequence {
                                tunnel: w633 -> [w643]
                                tunnel: [w642] -> w634
                                tunnel: w632 -> [w641]
                                tunnel: [w651] -> _
                                tunnel: w634 -> [w651]
                                frame #0 {
                                n175 = property on="odd/even indicator" class="Bool (strict)"() -> ("Value"=w640:bool)  [unwired: 2 in, 2 out]
                                n176 = case shown="True" w640 {
                                tunnel: [2 0] -> w646
                                tunnel: [2 0] -> w645
                                frame False {
                                }
                                frame True {
                                }
                                }
                                n177 = Index Array(array=w643, index (row)=w646, index (col)=w645) -> (element=w644:dbl)
                                n178 = call-poly <vilib>:"DAQmx Write.vi"("task/channels in"=w641, "data"=w644) -> ("task out"=w642:refnum<k21>)  [unwired: 11 in, 2 out]
                                }
                                frame #1 {
                                }
                                }
                                }
                                frame #2 {
                                n179 = for {
                                N: 9 -> [_]
                                tunnel: w654 -> [w673]
                                tunnel: w656 -> [w670]
                                tunnel: w661 -> [w671]
                                tunnel: w660 -> [w669]
                                tunnel: w653 -> [w672]
                                tunnel: [w671] -> w659
                                tunnel: [w670] -> w658
                                tunnel: [w669] -> w657
                                tunnel: w652 -> [w662]
                                i -> [w666]
                                n180 = property on="odd/even indicator" class="Bool (strict)"() -> ("Value"=w663:bool)  [unwired: 2 in, 2 out]
                                n181 = case shown="False" w663 {
                                tunnel: [i32[] [2, 2, 1, 1, 1, 0, 0, 0, 0, 2, 2, 2, 2, 2, 0] i32[] [0, 0, 1, 1, 1, 2, 2, 2, 2, 2, 2, 2, 2, 2, 0]] -> w668
                                tunnel: [i32[] [1, 0, 2, 1, 0, 2, 1, 0, 0, 0, 1, 2, 3, 4, 0] i32[] [1, 2, 0, 1, 2, 0, 1, 2, 2, 0, 1, 2, 3, 4, 0]] -> w667
                                frame False {
                                }
                                frame True {
                                }
                                }
                                n182 = flat-sequence {
                                tunnel: w673 -> [w682]
                                tunnel: w672 -> [w686]
                                tunnel: w671 -> [w685]
                                tunnel: w670 -> [w684]
                                tunnel: w669 -> [w683]
                                tunnel: w665 -> [w680]
                                tunnel: w664 -> [w679]
                                tunnel: w662 -> [w678]
                                frame #0 {
                                n183 = Index Array(array=w682, index (row)=w680, index (col)=w679) -> (element=w681:dbl)
                                n184 = call "take image.vi"("Voltage"=w681, "Exposure time"=w686, "expose any"=w678, "Busy out"=w683, "Exp In"=w684, "Galvo"=w685) -> ()  [unwired: 6 in]
                                }
                                frame #1 {
                                n185 = property on="Settle time" class="DigNum (strict)"() -> ("Value"=w687:u32)  [unwired: 2 in, 2 out]
                                n186 = Wait (ms)(milliseconds to wait=w687) -> ()  [unwired: 1 out]
                                }
                                }
                                n187 = Index Array(array=w667, index=w666) -> (element=w665:i32)
                                n188 = Index Array(array=w668, index=w666) -> (element=w664:i32)
                                }
                                }
                                frame #3 {
                                n189 = property on="acquire 488" class="Bool (strict)"() -> ("Value"=w691:bool)  [unwired: 2 in, 2 out]
                                n190 = property on="acquire 405" class="Bool (strict)"() -> ("Value"=w692:bool)  [unwired: 2 in, 2 out]
                                n191 = property on="acquire 640" class="Bool (strict)"() -> ("Value"=w690:bool)  [unwired: 2 in, 2 out]
                                n192 = Or(x=w691, y=w692) -> (x .or. y?=w689:bool)
                                n193 = Or(x=w689, y=w690) -> (x .or. y?=w688:bool)
                                n194 = case shown="False" w688 {
                                tunnel: w695 -> [_ w696]
                                frame False {
                                }
                                frame True {
                                n195 = call-poly <vilib>:"DAQmx Write.vi"("task/channels in"=w696, "data"=FALSE) -> ()  [unwired: 11 in, 3 out]
                                }
                                }
                                n196 = property on="odd/even indicator" class="Bool (strict)"() -> ("Value"=w694:bool)  [unwired: 2 in, 2 out]
                                n197 = Not(x=w694) -> (.not. x?=w693:bool)
                                n198 = property on="odd/even indicator" class="Bool (strict)"("Value"=w693) -> ()  [unwired: 2 in, 2 out]
                                }
                                }
                              }
                            }
                            n199 = case shown="True" "acquire 488" {
                              tunnel: w465 -> [w538 w544]
                              tunnel: w463 -> [w536 w548]
                              tunnel: w464 -> [w537 w549]
                              tunnel: [w538 w546] -> _
                              tunnel: [w537 w547] -> _
                              tunnel: [w536 w545] -> _
                              tunnel: w460 -> [_ _]
                              tunnel: w454 -> [_ w541]
                              tunnel: w457 -> [_ w540]
                              tunnel: w451 -> [_ w539]
                              frame False {
                              }
                              frame True {
                                n200 = property on="488 voltages" class="Arr (strict)"() -> ("Value"=w542:dbl[][])  [unwired: 2 in, 2 out]
                                n201 = stacked-sequence {
                                seq-local: [_ w558 _ _] -> [_ _ w579 _]
                                seq-local: [_ w557 _ _] -> [_ _ w578 _]
                                seq-local: [_ w556 _ _] -> [_ _ w574 _]
                                seq-local: [_ w555 _ _] -> [_ _ w572 _]
                                seq-local: [_ w554 _ _] -> [_ _ w571 _]
                                tunnel: w549 -> [_ w558 _ _]
                                tunnel: w548 -> [_ w557 _ _]
                                tunnel: w544 -> [_ w556 _ _]
                                tunnel: w542 -> [_ w555 _ _]
                                tunnel: "488 Exp" -> [_ w554 _ _]
                                tunnel: [_ _ w577 _] -> w547
                                tunnel: [_ _ w576 _] -> w546
                                tunnel: [_ _ w575 _] -> w545
                                tunnel: w542 -> [_ w553 _ _]
                                tunnel: w541 -> [_ w552 _ _]
                                tunnel: w540 -> [w550 _ _ w613]
                                tunnel: w539 -> [_ _ w570 _]
                                frame #0 {
                                n202 = call-poly <vilib>:"DAQmx Write.vi"("task/channels in"=w550, "data"=TRUE) -> ()  [unwired: 11 in, 3 out]
                                }
                                frame #1 {
                                n203 = flat-sequence {
                                tunnel: w553 -> [w565]
                                tunnel: w552 -> [w563]
                                tunnel: [w564] -> _
                                frame #0 {
                                n204 = property on="odd/even indicator" class="Bool (strict)"() -> ("Value"=w559:bool)  [unwired: 2 in, 2 out]
                                n205 = case shown="False" w559 {
                                tunnel: [2 0] -> w561
                                tunnel: [2 0] -> w560
                                frame False {
                                }
                                frame True {
                                }
                                }
                                n206 = Index Array(array=w565, index (row)=w561, index (col)=w560) -> (element=w562:dbl)
                                n207 = call-poly <vilib>:"DAQmx Write.vi"("task/channels in"=w563, "data"=w562) -> ("task out"=w564:refnum<k21>)  [unwired: 11 in, 2 out]
                                }
                                }
                                }
                                frame #2 {
                                n208 = for {
                                N: 9 -> [_]
                                tunnel: w572 -> [w591]
                                tunnel: w574 -> [w589]
                                tunnel: w579 -> [w590]
                                tunnel: w578 -> [w588]
                                tunnel: [w590] -> w577
                                tunnel: [w589] -> w576
                                tunnel: [w588] -> w575
                                tunnel: w571 -> [w587]
                                tunnel: w570 -> [w580]
                                i -> [w586]
                                n209 = property on="odd/even indicator" class="Bool (strict)"() -> ("Value"=w581:bool)  [unwired: 2 in, 2 out]
                                n210 = case shown="True" w581 {
                                tunnel: [i32[] [2, 2, 1, 1, 1, 0, 0, 0, 0, 2, 2, 2, 2, 2, 0] i32[] [0, 0, 1, 1, 1, 2, 2, 2, 2, 2, 2, 2, 2, 2, 0]] -> w582
                                tunnel: [i32[] [1, 0, 2, 1, 0, 2, 1, 0, 0, 0, 1, 2, 3, 4, 0] i32[] [1, 2, 0, 1, 2, 0, 1, 2, 2, 0, 1, 2, 3, 4, 0]] -> w583
                                frame False {
                                }
                                frame True {
                                }
                                }
                                n211 = Index Array(array=w583, index=w586) -> (element=w585:i32)
                                n212 = Index Array(array=w582, index=w586) -> (element=w584:i32)
                                n213 = flat-sequence {
                                tunnel: w591 -> [w600]
                                tunnel: w587 -> [w604]
                                tunnel: w590 -> [w603]
                                tunnel: w589 -> [w602]
                                tunnel: w588 -> [w601]
                                tunnel: w585 -> [w598]
                                tunnel: w584 -> [w597]
                                tunnel: w580 -> [w596]
                                frame #0 {
                                n214 = Index Array(array=w600, index (row)=w598, index (col)=w597) -> (element=w599:dbl)
                                n215 = call "take image.vi"("Voltage"=w599, "Exposure time"=w604, "expose any"=w596, "Busy out"=w601, "Exp In"=w602, "Galvo"=w603) -> ()  [unwired: 6 in]
                                }
                                frame #1 {
                                n216 = property on="Settle time" class="DigNum (strict)"() -> ("Value"=w605:u32)  [unwired: 2 in, 2 out]
                                n217 = Wait (ms)(milliseconds to wait=w605) -> ()  [unwired: 1 out]
                                }
                                }
                                }
                                }
                                frame #3 {
                                n218 = property on="acquire 561" class="Bool (strict)"() -> ("Value"=w609:bool)  [unwired: 2 in, 2 out]
                                n219 = property on="acquire 405" class="Bool (strict)"() -> ("Value"=w608:bool)  [unwired: 2 in, 2 out]
                                n220 = property on="acquire 640" class="Bool (strict)"() -> ("Value"=w610:bool)  [unwired: 2 in, 2 out]
                                n221 = property on="odd/even indicator" class="Bool (strict)"() -> ("Value"=w611:bool)  [unwired: 2 in, 2 out]
                                n222 = Not(x=w611) -> (.not. x?=w612:bool)
                                n223 = Or(x=w609, y=w608) -> (x .or. y?=w607:bool)
                                n224 = property on="odd/even indicator" class="Bool (strict)"("Value"=w612) -> ()  [unwired: 2 in, 2 out]
                                n225 = Or(x=w607, y=w610) -> (x .or. y?=w606:bool)
                                n226 = case shown="True" w606 {
                                tunnel: w613 -> [_ w614]
                                frame False {
                                }
                                frame True {
                                n227 = call-poly <vilib>:"DAQmx Write.vi"("task/channels in"=w614, "data"=FALSE) -> ()  [unwired: 11 in, 3 out]
                                }
                                }
                                }
                                }
                              }
                            }
                            n228 = case shown="True" "acquire 405" {
                              tunnel: w456 -> [_ w479]
                              tunnel: w454 -> [_ w477]
                              tunnel: w453 -> [_ w475]
                              tunnel: w452 -> [_ w474]
                              tunnel: w451 -> [_ w473]
                              frame False {
                              }
                              frame True {
                                n229 = property on="405 voltages" class="Arr (strict)"() -> ("Value"=w478:dbl[][])  [unwired: 2 in, 2 out]
                                n230 = stacked-sequence {
                                tunnel: w478 -> [_ w483 w498 _]
                                tunnel: w477 -> [_ w482 w497 _]
                                tunnel: [_ _ _ w533] -> _
                                tunnel: w479 -> [w480 _ _ w533]
                                tunnel: "405 Exp" -> [_ _ w496 _]
                                tunnel: w475 -> [_ _ w495 _]
                                tunnel: w474 -> [_ _ w494 _]
                                tunnel: w473 -> [_ _ w493 _]
                                frame #0 {
                                n231 = call-poly <vilib>:"DAQmx Write.vi"("task/channels in"=w480, "data"=TRUE) -> ()  [unwired: 11 in, 3 out]
                                }
                                frame #1 {
                                n232 = flat-sequence {
                                tunnel: w483 -> [w487]
                                tunnel: [w486] -> w484
                                tunnel: w482 -> [w485]
                                tunnel: [w492] -> _
                                tunnel: w484 -> [w492]
                                frame #0 {
                                n233 = Index Array(array=w487, index (row)=0, index (col)=0) -> (element=w488:dbl)
                                n234 = call-poly <vilib>:"DAQmx Write.vi"("task/channels in"=w485, "data"=w488) -> ("task out"=w486:refnum<k21>)  [unwired: 11 in, 2 out]
                                }
                                frame #1 {
                                n235 = Wait (ms)(milliseconds to wait=50) -> ()  [unwired: 1 out]
                                }
                                }
                                }
                                frame #2 {
                                n236 = for {
                                N: 9 -> [_]
                                tunnel: w498 -> [w509]
                                tunnel: w497 -> [w508]
                                tunnel: w496 -> [w507]
                                tunnel: w495 -> [w506]
                                tunnel: w494 -> [w505]
                                tunnel: w493 -> [w500]
                                i -> [w504]
                                n237 = property on="odd/even indicator" class="Bool (strict)"() -> ("Value"=w501:bool)  [unwired: 2 in, 2 out]
                                n238 = case shown="True" w501 {
                                tunnel: [i32[] [2, 2, 1, 1, 1, 0, 0, 0, 0, 2, 2, 2, 2, 2, 0] i32[] [0, 0, 1, 1, 1, 2, 2, 2, 2, 2, 2, 2, 2, 2, 0]] -> w503
                                tunnel: [i32[] [1, 0, 2, 1, 0, 2, 1, 0, 0, 0, 1, 2, 3, 4, 0] i32[] [1, 2, 0, 1, 2, 0, 1, 2, 2, 0, 1, 2, 3, 4, 0]] -> w502
                                frame False {
                                }
                                frame True {
                                }
                                }
                                n239 = flat-sequence {
                                tunnel: w511 -> [w523]
                                tunnel: w510 -> [w522]
                                tunnel: w509 -> [w521]
                                tunnel: w508 -> [w520]
                                tunnel: w507 -> [w519]
                                tunnel: w506 -> [w518]
                                tunnel: w505 -> [w517]
                                tunnel: w500 -> [w516]
                                frame #0 {
                                n240 = Index Array(array=w521, index (row)=w523, index (col)=w522) -> (element=w524:dbl)
                                n241 = call "take image.vi"("Voltage"=w524, "Exposure time"=w519, "expose any"=w516, "Busy out"=w517, "Exp In"=w518, "Galvo"=w520) -> ()  [unwired: 6 in]
                                }
                                frame #1 {
                                n242 = property on="Settle time" class="DigNum (strict)"() -> ("Value"=w525:u32)  [unwired: 2 in, 2 out]
                                n243 = Wait (ms)(milliseconds to wait=w525) -> ()  [unwired: 1 out]
                                }
                                }
                                n244 = Index Array(array=w502, index=w504) -> (element=w511:i32)
                                n245 = Index Array(array=w503, index=w504) -> (element=w510:i32)
                                }
                                }
                                frame #3 {
                                n246 = property on="acquire 561" class="Bool (strict)"() -> ("Value"=w528:bool)  [unwired: 2 in, 2 out]
                                n247 = property on="acquire 488" class="Bool (strict)"() -> ("Value"=w529:bool)  [unwired: 2 in, 2 out]
                                n248 = property on="acquire 640" class="Bool (strict)"() -> ("Value"=w527:bool)  [unwired: 2 in, 2 out]
                                n249 = Or(x=w528, y=w529) -> (x .or. y?=w530:bool)
                                n250 = property on="odd/even indicator" class="Bool (strict)"() -> ("Value"=w532:bool)  [unwired: 2 in, 2 out]
                                n251 = Or(x=w530, y=w527) -> (x .or. y?=w526:bool)
                                n252 = Not(x=w532) -> (.not. x?=w531:bool)
                                n253 = property on="odd/even indicator" class="Bool (strict)"("Value"=w531) -> ()  [unwired: 2 in, 2 out]
                                n254 = case shown="True" w526 {
                                tunnel: w533 -> [_ w534]
                                frame False {
                                }
                                frame True {
                                n255 = call-poly <vilib>:"DAQmx Write.vi"("task/channels in"=w534, "data"=FALSE) -> ()  [unwired: 11 in, 3 out]
                                }
                                }
                                }
                                }
                              }
                            }
                          }
                          frame "fast sequence" {
                            # "561"
                            # "488"
                            # "fast sequence"
                            n256 = property on="647 Exp" class="DigNum (strict)"() -> ("Value"=w784:dbl)  [unwired: 2 in, 2 out]
                            n257 = property on="647 voltages" class="Arr (strict)"() -> ("Value"=w787:dbl[][])  [unwired: 2 in, 2 out]
                            n258 = stacked-sequence {
                              seq-local: [_ w869 _ _] -> [_ _ w887 _]
                              seq-local: [_ w868 _ _] -> [_ _ w886 _]
                              seq-local: [_ w867 _ _] -> [_ _ w885 _]
                              seq-local: [_ w866 _ _] -> [_ _ w881 _]
                              seq-local: [_ w865 _ _] -> [_ _ w880 _]
                              tunnel: w795 -> [_ w869 _ _]
                              tunnel: w790 -> [_ w868 _ _]
                              tunnel: w794 -> [_ w867 _ _]
                              tunnel: w787 -> [_ w866 _ _]
                              tunnel: w784 -> [_ w865 _ _]
                              tunnel: [_ _ w884 _] -> w792
                              tunnel: [_ _ w883 _] -> w791
                              tunnel: [_ _ w882 _] -> w793
                              tunnel: w787 -> [_ w863 _ _]
                              tunnel: w790 -> [_ w862 _ _]
                              tunnel: w789 -> [w860 _ _ w918]
                              tunnel: w783 -> [w858 _ _ w916]
                              tunnel: w781 -> [_ _ w878 _]
                              frame #0 {
                                n259 = VISA Write(VISA resource name=w860, write buffer="la on\r" ("format string")) -> ()  [unwired: 1 in, 3 out]
                                n260 = call-poly <vilib>:"DAQmx Write.vi"("task/channels in"=w858, "data"=TRUE) -> ()  [unwired: 11 in, 3 out]
                              }
                              frame #1 {
                                n261 = flat-sequence {
                                tunnel: [w870] -> _
                                tunnel: w863 -> [w872]
                                tunnel: [w871] -> w864
                                tunnel: w862 -> [w870]
                                tunnel: [w877] -> _
                                tunnel: w864 -> [w877]
                                frame #0 {
                                n262 = Index Array(array=w872, index (row)=0, index (col)=0) -> (element=w873:dbl)
                                n263 = call-poly <vilib>:"DAQmx Write.vi"("task/channels in"=w870, "data"=w873) -> ("task out"=w871:refnum<k21>)  [unwired: 11 in, 2 out]
                                }
                                frame #1 {
                                n264 = Wait (ms)(milliseconds to wait=50) -> ()  [unwired: 1 out]
                                }
                                }
                              }
                              frame #2 {
                                n265 = for {
                                N: 9 -> [_]
                                tunnel: w881 -> [w899]
                                tunnel: w887 -> [w896]
                                tunnel: w886 -> [w897]
                                tunnel: w885 -> [w895]
                                tunnel: w880 -> [w898]
                                tunnel: [w897] -> w884
                                tunnel: [w896] -> w883
                                tunnel: [w895] -> w882
                                tunnel: w878 -> [w888]
                                i -> [w893]
                                n266 = property on="odd/even indicator" class="Bool (strict)"() -> ("Value"=w891:bool)  [unwired: 2 in, 2 out]
                                n267 = case shown="False" w891 {
                                tunnel: [i32[] [2, 2, 1, 1, 1, 0, 0, 0, 0, 2, 2, 2, 2, 2, 0] i32[] [0, 0, 1, 1, 1, 2, 2, 2, 2, 2, 2, 2, 2, 2, 0]] -> w889
                                tunnel: [i32[] [1, 0, 2, 1, 0, 2, 1, 0, 0, 0, 1, 2, 3, 4, 0] i32[] [1, 2, 0, 1, 2, 0, 1, 2, 2, 0, 1, 2, 3, 4, 0]] -> w890
                                frame False {
                                }
                                frame True {
                                }
                                }
                                n268 = Index Array(array=w890, index=w893) -> (element=w894:i32)
                                n269 = flat-sequence {
                                tunnel: w899 -> [w908]
                                tunnel: w898 -> [w912]
                                tunnel: w897 -> [w911]
                                tunnel: w896 -> [w910]
                                tunnel: w895 -> [w909]
                                tunnel: w892 -> [w906]
                                tunnel: w894 -> [w905]
                                tunnel: w888 -> [w904]
                                frame #0 {
                                n270 = Index Array(array=w908, index (row)=w905, index (col)=w906) -> (element=w907:dbl)
                                n271 = call "take image.vi"("Voltage"=w907, "Exposure time"=w912, "expose any"=w904, "Busy out"=w909, "Exp In"=w910, "Galvo"=w911) -> ()  [unwired: 6 in]
                                }
                                frame #1 {
                                n272 = property on="Settle time" class="DigNum (strict)"() -> ("Value"=w913:u32)  [unwired: 2 in, 2 out]
                                n273 = Wait (ms)(milliseconds to wait=w913) -> ()  [unwired: 1 out]
                                }
                                }
                                n274 = Index Array(array=w889, index=w893) -> (element=w892:i32)
                                }
                              }
                              frame #3 {
                                n275 = property on="odd/even indicator" class="Bool (strict)"() -> ("Value"=w914:bool)  [unwired: 2 in, 2 out]
                                n276 = Not(x=w914) -> (.not. x?=w915:bool)
                                n277 = property on="odd/even indicator" class="Bool (strict)"("Value"=w915) -> ()  [unwired: 2 in, 2 out]
                                n278 = VISA Write(VISA resource name=w918, write buffer="la off\r" ("format string")) -> ()  [unwired: 1 in, 3 out]
                                n279 = call-poly <vilib>:"DAQmx Write.vi"("task/channels in"=w916, "data"=FALSE) -> ()  [unwired: 11 in, 3 out]
                              }
                            }
                            n280 = property on="561 voltages" class="Arr (strict)"() -> ("Value"=w786:dbl[][])  [unwired: 2 in, 2 out]
                            n281 = property on="561 Exp" class="DigNum (strict)"() -> ("Value"=w785:dbl)  [unwired: 2 in, 2 out]
                            n282 = stacked-sequence {
                              seq-local: [_ w807 _ _] -> [_ _ w825 _]
                              seq-local: [_ w806 _ _] -> [_ _ w824 _]
                              seq-local: [_ w805 _ _] -> [_ _ w820 _]
                              seq-local: [_ w804 _ _] -> [_ _ w818 _]
                              seq-local: [_ w803 _ _] -> [_ _ w817 _]
                              tunnel: w792 -> [_ w807 _ _]
                              tunnel: w793 -> [_ w806 _ _]
                              tunnel: w791 -> [_ w805 _ _]
                              tunnel: w786 -> [_ w804 _ _]
                              tunnel: w785 -> [_ w803 _ _]
                              tunnel: [_ _ w823 _] -> _
                              tunnel: [_ _ w822 _] -> _
                              tunnel: [_ _ w821 _] -> _
                              tunnel: w786 -> [_ w801 _ _]
                              tunnel: w790 -> [_ w800 _ _]
                              tunnel: w788 -> [w799 _ _ w856]
                              tunnel: w782 -> [w796 _ _ w854]
                              tunnel: w781 -> [_ _ w816 _]
                              frame #0 {
                                n283 = call-poly <vilib>:"DAQmx Write.vi"("task/channels in"=w799, "data"=TRUE) -> ()  [unwired: 11 in, 3 out]
                                n284 = call-poly <vilib>:"DAQmx Write.vi"("task/channels in"=w796, "data"=TRUE) -> ()  [unwired: 11 in, 3 out]
                              }
                              frame #1 {
                                n285 = flat-sequence {
                                tunnel: w801 -> [w810]
                                tunnel: [w809] -> w802
                                tunnel: w800 -> [w808]
                                tunnel: [w815] -> _
                                tunnel: w802 -> [w815]
                                frame #0 {
                                n286 = Index Array(array=w810, index (row)=0, index (col)=0) -> (element=w811:dbl)
                                n287 = call-poly <vilib>:"DAQmx Write.vi"("task/channels in"=w808, "data"=w811) -> ("task out"=w809:refnum<k21>)  [unwired: 11 in, 2 out]
                                }
                                frame #1 {
                                n288 = Wait (ms)(milliseconds to wait=50) -> ()  [unwired: 1 out]
                                }
                                }
                              }
                              frame #2 {
                                n289 = for {
                                N: 9 -> [_]
                                tunnel: w818 -> [w837]
                                tunnel: w820 -> [w834]
                                tunnel: w825 -> [w835]
                                tunnel: w824 -> [w833]
                                tunnel: w817 -> [w836]
                                tunnel: [w835] -> w823
                                tunnel: [w834] -> w822
                                tunnel: [w833] -> w821
                                tunnel: w816 -> [w826]
                                i -> [w832]
                                n290 = property on="odd/even indicator" class="Bool (strict)"() -> ("Value"=w827:bool)  [unwired: 2 in, 2 out]
                                n291 = case shown="True" w827 {
                                tunnel: [i32[] [2, 2, 1, 1, 1, 0, 0, 0, 0, 2, 2, 2, 2, 2, 0] i32[] [0, 0, 1, 1, 1, 2, 2, 2, 2, 2, 2, 2, 2, 2, 0]] -> w828
                                tunnel: [i32[] [1, 0, 2, 1, 0, 2, 1, 0, 0, 0, 1, 2, 3, 4, 0] i32[] [1, 2, 0, 1, 2, 0, 1, 2, 2, 0, 1, 2, 3, 4, 0]] -> w829
                                frame False {
                                }
                                frame True {
                                }
                                }
                                n292 = Index Array(array=w829, index=w832) -> (element=w831:i32)
                                n293 = Index Array(array=w828, index=w832) -> (element=w830:i32)
                                n294 = flat-sequence {
                                tunnel: w837 -> [w846]
                                tunnel: w836 -> [w850]
                                tunnel: w835 -> [w849]
                                tunnel: w834 -> [w848]
                                tunnel: w833 -> [w847]
                                tunnel: w831 -> [w844]
                                tunnel: w830 -> [w843]
                                tunnel: w826 -> [w842]
                                frame #0 {
                                n295 = Index Array(array=w846, index (row)=w844, index (col)=w843) -> (element=w845:dbl)
                                n296 = call "take image.vi"("Voltage"=w845, "Exposure time"=w850, "expose any"=w842, "Busy out"=w847, "Exp In"=w848, "Galvo"=w849) -> ()  [unwired: 6 in]
                                }
                                frame #1 {
                                n297 = property on="Settle time" class="DigNum (strict)"() -> ("Value"=w851:u32)  [unwired: 2 in, 2 out]
                                n298 = Wait (ms)(milliseconds to wait=w851) -> ()  [unwired: 1 out]
                                }
                                }
                                }
                              }
                              frame #3 {
                                n299 = call-poly <vilib>:"DAQmx Write.vi"("task/channels in"=w856, "data"=FALSE) -> ()  [unwired: 11 in, 3 out]
                                n300 = property on="odd/even indicator" class="Bool (strict)"() -> ("Value"=w853:bool)  [unwired: 2 in, 2 out]
                                n301 = call-poly <vilib>:"DAQmx Write.vi"("task/channels in"=w854, "data"=FALSE) -> ()  [unwired: 11 in, 3 out]
                                n302 = Not(x=w853) -> (.not. x?=w852:bool)
                                n303 = property on="odd/even indicator" class="Bool (strict)"("Value"=w852) -> ()  [unwired: 2 in, 2 out]
                              }
                            }
                          }
                          frame "optosplit" {
                            n304 = case shown="False" w921 {
                              tunnel: w924 -> [w930 w967]
                              tunnel: w923 -> [w929 w966]
                              tunnel: w922 -> [w928 w965]
                              tunnel: w920 -> [_ w959]
                              frame True {
                                w925 = 15
                                # "With optosplit"
                                n305 = flat-sequence {
                                tunnel: w928 -> [w934]
                                tunnel: w927 -> [w933]
                                tunnel: [w932] -> w931
                                tunnel: [w941] -> w926
                                tunnel: w931 -> [w941]
                                frame #0 {
                                n306 = Index Array(array=w933, index (row)=0, index (col)=0) -> (element=w935:dbl)
                                n307 = call-poly <vilib>:"DAQmx Write.vi"("task/channels in"=w934, "data"=w935) -> ("task out"=w932:refnum<k21>)  [unwired: 11 in, 2 out]
                                }
                                frame #1 {
                                n308 = property on="Settle time" class="DigNum (strict)"() -> ("Value"=w940:u32)  [unwired: 2 in, 2 out]
                                n309 = Add(x=w940, y=20) -> (x+y=w939:u32)
                                n310 = Wait (ms)(milliseconds to wait=w939) -> ()  [unwired: 1 out]
                                }
                                }
                                n311 = property on="561 voltages" class="Arr (strict)"() -> ("Value"=w927:dbl[][])  [unwired: 2 in, 2 out]
                                n312 = for {
                                N: w925 -> [_]
                                tunnel: w927 -> [w949]
                                tunnel: w930 -> [w952]
                                tunnel: w929 -> [w951]
                                tunnel: w926 -> [w950]
                                tunnel: w925 -> [_]
                                i -> [w945]
                                n313 = property on="Exposure time" class="DigNum (strict)"() -> ("Value"=w948:dbl)  [unwired: 2 in, 2 out]
                                n314 = Index Array(array=i32[] [1, 2, 3, 4, 0, 1, 2, 3, 4, 0, 1, 2, 3, 4, 0], index=w945) -> (element=w943:i32)
                                n315 = Index Array(array=i32[] [0, 0, 0, 0, 1, 1, 1, 1, 1, 2, 2, 2, 2, 2, 0], index=w945) -> (element=w944:i32)
                                n316 = Index Array(array=w949, index (row)=w943, index (col)=w944) -> (element=w942:dbl)
                                n317 = property on="Current voltage" class="DigNum (strict)"("Value"=w942) -> ()  [unwired: 2 in, 2 out]
                                n318 = flat-sequence {
                                tunnel: w952 -> [w957]
                                tunnel: w951 -> [w956]
                                tunnel: w942 -> [w955]
                                tunnel: w950 -> [w954]
                                tunnel: w948 -> [w953]
                                frame #0 {
                                n319 = call "take image.vi"("Voltage"=w955, "Exposure time"=w953, "Busy out"=w956, "Exp In"=w957, "Galvo"=w954) -> ()  [unwired: 7 in]
                                }
                                frame #1 {
                                n320 = property on="Settle time" class="DigNum (strict)"() -> ("Value"=w958:u32)  [unwired: 2 in, 2 out]
                                n321 = Wait (ms)(milliseconds to wait=w958) -> ()  [unwired: 1 out]
                                }
                                }
                                }
                              }
                              frame False {
                                w962 = 9
                                # "With optosplit"
                                n322 = flat-sequence {
                                tunnel: w965 -> [w974]
                                tunnel: w964 -> [w973]
                                tunnel: [w972] -> w968
                                tunnel: [w983] -> w963
                                tunnel: w968 -> [w983]
                                frame #0 {
                                n323 = property on="odd/even indicator" class="Bool (strict)"() -> ("Value"=w971:bool)  [unwired: 2 in, 2 out]
                                n324 = case shown="False" w971 {
                                tunnel: [2 0] -> w970
                                tunnel: [2 0] -> w969
                                frame False {
                                }
                                frame True {
                                }
                                }
                                n325 = Index Array(array=w973, index (row)=w970, index (col)=w969) -> (element=w975:dbl)
                                n326 = call-poly <vilib>:"DAQmx Write.vi"("task/channels in"=w974, "data"=w975) -> ("task out"=w972:refnum<k21>)  [unwired: 11 in, 2 out]
                                }
                                frame #1 {
                                n327 = property on="Settle time" class="DigNum (strict)"() -> ("Value"=w982:u32)  [unwired: 2 in, 2 out]
                                n328 = Add(x=w982, y=20) -> (x+y=w981:u32)
                                n329 = Wait (ms)(milliseconds to wait=w981) -> ()  [unwired: 1 out]
                                }
                                }
                                n330 = property on="561 voltages" class="Arr (strict)"() -> ("Value"=w964:dbl[][])  [unwired: 2 in, 2 out]
                                n331 = for {
                                N: w962 -> [_]
                                tunnel: w964 -> [w993]
                                tunnel: w967 -> [w996]
                                tunnel: w966 -> [w995]
                                tunnel: w963 -> [w994]
                                tunnel: w962 -> [_]
                                tunnel: [w985] -> w960
                                tunnel: w959 -> [w984]
                                i -> [w991]
                                n332 = property on="odd/even indicator" class="Bool (strict)"() -> ("Value"=w985:bool)  [unwired: 2 in, 2 out]
                                n333 = property on="Exposure time" class="DigNum (strict)"() -> ("Value"=w992:dbl)  [unwired: 2 in, 2 out]
                                n334 = case shown="False" w985 {
                                tunnel: [i32[] [2, 2, 1, 1, 1, 0, 0, 0, 0, 2, 2, 2, 2, 2, 0] i32[] [0, 0, 1, 1, 1, 2, 2, 2, 2, 2, 2, 2, 2, 2, 0]] -> w986
                                tunnel: [i32[] [1, 0, 2, 1, 0, 2, 1, 0, 0, 0, 1, 2, 3, 4, 0] i32[] [1, 2, 0, 1, 2, 0, 1, 2, 2, 0, 1, 2, 3, 4, 0]] -> w987
                                frame False {
                                }
                                frame True {
                                }
                                }
                                n335 = Index Array(array=w987, index=w991) -> (element=w989:i32)
                                n336 = Index Array(array=w986, index=w991) -> (element=w990:i32)
                                n337 = Index Array(array=w993, index (row)=w989, index (col)=w990) -> (element=w988:dbl)
                                n338 = property on="Current voltage" class="DigNum (strict)"("Value"=w988) -> ()  [unwired: 2 in, 2 out]
                                n339 = flat-sequence {
                                tunnel: w996 -> [w1006]
                                tunnel: w995 -> [w1005]
                                tunnel: w988 -> [w1004]
                                tunnel: w994 -> [w1003]
                                tunnel: w992 -> [w1002]
                                tunnel: w984 -> [w1001]
                                frame #0 {
                                n340 = call "take image.vi"("Voltage"=w1004, "Exposure time"=w1002, "expose any"=w1001, "Busy out"=w1005, "Exp In"=w1006, "Galvo"=w1003) -> ()  [unwired: 6 in]
                                }
                                frame #1 {
                                n341 = property on="Settle time" class="DigNum (strict)"() -> ("Value"=w1007:u32)  [unwired: 2 in, 2 out]
                                n342 = Wait (ms)(milliseconds to wait=w1007) -> ()  [unwired: 1 out]
                                }
                                }
                                }
                                n343 = Not(x=w960) -> (.not. x?=w961:bool)
                                n344 = property on="odd/even indicator" class="Bool (strict)"("Value"=w961) -> ()  [unwired: 2 in, 2 out]
                              }
                            }
                          }
                          frame "rolling SIM" {
                            w1011 = 0 ("index")
                            # "Rolling SIM"
                            n345 = Build Array("short delay", "short delay", "long delay") -> (w1012:dbl[])
                            n346 = Insert Into Array(array=w1012, index=w1011, new element=w1012) -> (w1013:dbl[])
                            n347 = Insert Into Array(array=w1013, index=w1011, new element=w1013) -> (w1008:dbl[])
                            n348 = property on="561 voltages" class="Arr (strict)"() -> ("Value"=w1019:dbl[][])  [unwired: 2 in, 2 out]
                            n349 = for {
                              N: 12 -> [_]
                              tunnel: w1019 -> [w1024]
                              tunnel: w1021 -> [w1035]
                              tunnel: w1020 -> [w1034]
                              tunnel: [w1027] -> w1016
                              tunnel: w1015 -> [w1026]
                              tunnel: w1014 -> [w1025]
                              tunnel: w1008 -> [w1022] mode=indexing
                              i -> [w1023]
                              n350 = property on="Exposure time" class="DigNum (strict)"() -> ("Value"=w1033:dbl)  [unwired: 2 in, 2 out]
                              n351 = Index Array(array=i32[] [1, 2, 0, 1, 2, 0, 1, 2, 2, 1, 0, 0, 3, 4, 0], index=w1023) -> (element=w1031:i32)
                              n352 = Index Array(array=i32[] [0, 0, 1, 1, 1, 2, 2, 2, 1, 1, 1, 0, 2, 2, 0], index=w1023) -> (element=w1032:i32)
                              n353 = Index Array(array=w1024, index (row)=w1031, index (col)=w1032) -> (element=w1030:dbl)
                              n354 = property on="Current voltage" class="DigNum (strict)"("Value"=w1030) -> ()  [unwired: 2 in, 2 out]
                              n355 = flat-sequence {
                                tunnel: w1035 -> [w1041]
                                tunnel: w1034 -> [w1037]
                                tunnel: w1030 -> [w1040]
                                tunnel: w1033 -> [w1039]
                                tunnel: w1026 -> [w1038]
                                tunnel: w1025 -> [w1036]
                                tunnel: w1022 -> [w1042]
                                frame #0 {
                                n356 = call "take image.vi"("Voltage"=w1040, "Exposure time"=w1039, "expose any"=w1038, "Busy out"=w1037, "Exp In"=w1041, "Galvo"=w1036) -> ()  [unwired: 6 in]
                                }
                                frame #1 {
                                n357 = Wait (ms)(milliseconds to wait=w1042) -> ()  [unwired: 1 out]
                                }
                              }
                              n358 = property on="odd/even indicator" class="Bool (strict)"() -> ("Value"=w1027:bool)  [unwired: 2 in, 2 out]
                            }
                            n359 = Not(x=w1016) -> (.not. x?=w1017:bool)
                            n360 = property on="odd/even indicator" class="Bool (strict)"("Value"=w1017) -> ()  [unwired: 2 in, 2 out]
                          }
                        }
                      }
                      frame #1 {
                        n361 = Greater?(x=w1046, y=1) -> (0:w1045:bool)
                        n362 = Greater?(x="Steps /um", y=0) -> (0:w1044:bool)
                        n363 = And(x=w1045, y=w1044) -> (x .and. y?=w1043:bool)
                        n364 = case shown="True" w1043 {
                          tunnel: w1051 -> [w1052 w1055]
                          tunnel: [w1052 w1054] -> w1050
                          tunnel: "Steps /um" -> [_ w1053]
                          frame False {
                          }
                          frame True {
                            n365 = flat-sequence {
                              tunnel: w1055 -> [w1063]
                              tunnel: [w1062] -> w1056
                              tunnel: w1053 -> [w1059]
                              tunnel: [w1066] -> w1054
                              tunnel: w1056 -> [w1066]
                              frame #0 {
                                n366 = Multiply(x=w1059, y=10.0) -> (x*y=w1057:dbl)
                                n367 = Format Into String "Format Into String"(format string="movrel\\sz=%f\\s\\r\\n", w1057) -> (resulting string=w1060:string)  [unwired: 2 in, 1 out]
                                "resulting string" <- w1060
                                n368 = VISA Write(VISA resource name=w1063, write buffer=w1060) -> (VISA resource name out=w1062:refnum<visa-resource-name>, error out=→"optosplit stage error":errorcluster)  [unwired: 1 in, 1 out]
                              }
                              frame #1 {
                                n369 = Wait (ms)(milliseconds to wait=20) -> ()  [unwired: 1 out]
                              }
                            }
                          }
                        }
                      }
                    }
                  }
                }
                frame #1 {
                  n370 = flat-sequence {
                    tunnel: w1082 -> [w1092]
                    tunnel: w1081 -> [w1091]
                    tunnel: w1080 -> [w1090]
                    tunnel: w1079 -> [w1089]
                    tunnel: [w1088] -> w1076
                    tunnel: [w1087] -> w1073
                    tunnel: [w1086] -> w1070
                    tunnel: [w1085] -> w1069
                    tunnel: w1083 -> [w1116]
                    tunnel: [w1115] -> w1077
                    tunnel: w1076 -> [w1115]
                    tunnel: [w1114] -> w1074
                    tunnel: w1073 -> [w1114]
                    tunnel: [w1113] -> w1071
                    tunnel: w1070 -> [w1113]
                    tunnel: w1069 -> [w1112]
                    tunnel: [w1112] -> w1067
                    tunnel: [w1130] -> w1078
                    tunnel: w1077 -> [w1130]
                    tunnel: [w1129] -> w1075
                    tunnel: w1074 -> [w1129]
                    tunnel: [w1128] -> w1072
                    tunnel: w1071 -> [w1128]
                    tunnel: [w1127] -> w1068
                    tunnel: w1067 -> [w1127]
                    tunnel: w1078 -> [w1137]
                    tunnel: w1075 -> [w1136]
                    tunnel: w1072 -> [w1135]
                    tunnel: w1068 -> [w1134]
                    frame #0 {
                      n371 = case shown="False" FALSE {
                        tunnel: w1092 -> [w1096 w1104]
                        tunnel: w1091 -> [w1095 w1103]
                        tunnel: w1090 -> [w1094 w1102]
                        tunnel: w1089 -> [w1093 w1101]
                        tunnel: [w1093 w1100] -> w1088
                        tunnel: [w1094 w1099] -> w1087
                        tunnel: [w1095 w1098] -> w1086
                        tunnel: [w1096 w1097] -> w1085
                        frame False {
                        }
                        frame True {
                          n372 = call-poly <vilib>:"DAQmx Write.vi"("task/channels in"=w1103, "data"=FALSE) -> ("task out"=w1098:refnum<k21>)  [unwired: 11 in, 2 out]
                          n373 = call-poly <vilib>:"DAQmx Write.vi"("task/channels in"=w1104, "data"=FALSE) -> ("task out"=w1097:refnum<k21>)  [unwired: 11 in, 2 out]
                          n374 = call-poly <vilib>:"DAQmx Write.vi"("task/channels in"=w1102, "data"=FALSE) -> ("task out"=w1099:refnum<k21>)  [unwired: 11 in, 2 out]
                          n375 = VISA Write(VISA resource name=w1101, write buffer="la off\r" ("format string")) -> (VISA resource name out=w1100:refnum<visa-resource-name>)  [unwired: 1 in, 2 out]
                        }
                      }
                    }
                    frame #1 {
                      n376 = property on="z-slices" class="DigNum (strict)"() -> ("Value"=w1110:dbl)  [unwired: 2 in, 2 out]
                      n377 = property on="Optosplit" class="RadioBtnsControl (strict)" props=["Value"]() -> ()  [unwired: 2 in, 3 out]
                      n378 = Greater?(x=w1110, y=1) -> (0:w1109:bool)
                      n379 = case shown="False" w1109 {
                        tunnel: w1116 -> [_ w1123]
                        frame False {
                        }
                        frame True {
                          n380 = property on="z-slices" class="DigNum (strict)"() -> ("Value"=w1121:dbl)  [unwired: 2 in, 2 out]
                          n381 = property on="Steps /um" class="DigNum (strict)"() -> ("Value"=w1122:dbl)  [unwired: 2 in, 2 out]
                          n382 = Negate(x=w1122) -> (-x=w1120:dbl)
                          n383 = Multiply(x=w1120, y=w1121) -> (x*y=w1119:dbl)
                          n384 = Multiply(x=w1119, y=10.0) -> (x*y=w1117:dbl)
                          n385 = Format Into String "Format Into String"(format string="movrel\\sz=%f\\s\\r\\n", w1117) -> (resulting string=w1125:string)  [unwired: 2 in, 1 out]
                          "resulting string 2" <- w1125
                          n386 = VISA Write(VISA resource name=w1123, write buffer=w1125) -> (error out=→"stage error":errorcluster)  [unwired: 1 in, 2 out]
                        }
                      }
                    }
                    frame #2 {
                      n387 = Multiply(x="interval /s", y=1000.0) -> (x*y=w1133:dbl)
                      n388 = Wait (ms)(milliseconds to wait=w1133) -> ()  [unwired: 1 out]
                    }
                    frame #3 {
                      n389 = property on="Optosplit" class="RadioBtnsControl (strict)"() -> ("Value"=w1138:T2)  [unwired: 2 in, 2 out]
                      n390 = disable-structure shown="Disabled" {
                        disable-tunnel: w1138 -> [w1143 _]
                        disable-tunnel: w1137 -> [w1142 _]
                        disable-tunnel: w1136 -> [w1141 _]
                        disable-tunnel: w1135 -> [w1140 _]
                        disable-tunnel: w1134 -> [w1139 _]
                        frame Disabled {
                          n391 = case shown="\"rolling SIM\"" w1143 {
                            tunnel: w1142 -> [_ w1147 w1155 w1163]
                            tunnel: w1141 -> [_ w1146 w1154 w1162]
                            tunnel: w1140 -> [_ w1145 w1153 w1161]
                            tunnel: w1139 -> [_ w1144 w1152 w1160]
                            frame "sequential", Default {
                            }
                            frame "optosplit" {
                              n392 = call-poly <vilib>:"DAQmx Write.vi"("task/channels in"=w1145, "data"=TRUE) -> ()  [unwired: 11 in, 3 out]
                              n393 = call-poly <vilib>:"DAQmx Write.vi"("task/channels in"=w1144, "data"=TRUE) -> ()  [unwired: 11 in, 3 out]
                              n394 = call-poly <vilib>:"DAQmx Write.vi"("task/channels in"=w1146, "data"=TRUE) -> ()  [unwired: 11 in, 3 out]
                              n395 = VISA Write(VISA resource name=w1147, write buffer="la on\r" ("format string")) -> ()  [unwired: 1 in, 3 out]
                            }
                            frame "rolling SIM" {
                              n396 = call-poly <vilib>:"DAQmx Write.vi"("task/channels in"=w1153, "data"=TRUE) -> ()  [unwired: 11 in, 3 out]
                              n397 = call-poly <vilib>:"DAQmx Write.vi"("task/channels in"=w1152, "data"=TRUE) -> ()  [unwired: 11 in, 3 out]
                              n398 = call-poly <vilib>:"DAQmx Write.vi"("task/channels in"=w1154, "data"=TRUE) -> ()  [unwired: 11 in, 3 out]
                              n399 = VISA Write(VISA resource name=w1155, write buffer="la on\r" ("format string")) -> ()  [unwired: 1 in, 3 out]
                            }
                            frame "fast sequence" {
                              n400 = call-poly <vilib>:"DAQmx Write.vi"("task/channels in"=w1161, "data"=TRUE) -> ()  [unwired: 11 in, 3 out]
                              n401 = call-poly <vilib>:"DAQmx Write.vi"("task/channels in"=w1160, "data"=TRUE) -> ()  [unwired: 11 in, 3 out]
                              n402 = call-poly <vilib>:"DAQmx Write.vi"("task/channels in"=w1162, "data"=TRUE) -> ()  [unwired: 11 in, 3 out]
                              n403 = VISA Write(VISA resource name=w1163, write buffer="la on\r" ("format string")) -> ()  [unwired: 1 in, 3 out]
                            }
                          }
                        }
                        frame Enabled {
                        }
                      }
                    }
                  }
                }
              }
              n404 = property on="Go SIM" class="Bool (strict)"() -> ("Value"=w383:bool)  [unwired: 2 in, 2 out]
              n405 = Not(x=w383) -> (.not. x?=w382:bool)
            }
          }
          frame #3 {
            w1170 = FALSE
            n406 = property on="Go SIM" class="Bool (strict)"("Value"=FALSE ("Go SIM")) -> ()  [unwired: 2 in, 2 out]
            n407 = property on="Tab Control" class="TabCtl (strict)"("DisabledEnum"=T4."Enabled" ("Disabled")) -> ()  [unwired: 2 in, 2 out]
            n408 = call-poly <vilib>:"DAQmx Write.vi"("task/channels in"=w1173, "data"=FALSE) -> ()  [unwired: 11 in, 3 out]
            n409 = call-poly <vilib>:"DAQmx Write.vi"("task/channels in"=w1174, "data"=FALSE) -> ()  [unwired: 11 in, 3 out]
            n410 = VISA Write(VISA resource name=w1171, write buffer="la off\r" ("format string")) -> ()  [unwired: 1 in, 3 out]
            n411 = property on="561" class="Bool (strict)"("Value"=w1170) -> ()  [unwired: 2 in, 2 out]
            n412 = property on="488" class="Bool (strict)"("Value"=w1170) -> ()  [unwired: 2 in, 2 out]
            n413 = property on="405" class="Bool (strict)"("Value"=w1170) -> ()  [unwired: 2 in, 2 out]
            n414 = property on="647" class="Bool (strict)"("Value"=w1170) -> ()  [unwired: 2 in, 2 out]
          }
        }
      }
    }
    n415 = property on="stop" class="Bool (strict)"() -> ("Value"=w209:bool)  [unwired: 2 in, 2 out]
    n416 = Wait (ms)(milliseconds to wait=u32 100) -> ()  [unwired: 1 out]
  }
  n417 = VISA Write(VISA resource name=w34, write buffer="en 1\r" ("format string")) -> (VISA resource name out=w33:refnum<visa-resource-name>)  [unwired: 1 in, 2 out]
  n418 = while {
    tunnel: w75 -> [w1187]
    tunnel: w76 -> [w1188]
    tunnel: [w1188] -> w65
    tunnel: [w1187] -> w64
    tunnel: w33 -> [w1182]
    tunnel: w32 -> [w1185]
    tunnel: [w1184] -> w45
    tunnel: [w1183] -> w44
    tunnel: w7 -> [w1180]
    tunnel: [w1180] -> w6
    tunnel: w1 -> [w1178]
    stop <- w1186 stop-if-true
    w1179 = 100
    n419 = Wait (ms)(milliseconds to wait=u32 250) -> ()  [unwired: 1 out]
    n420 = event shown="[1] \"Jog Z\": Value Change" {
      selector: _ -> [_ _]
      dyn-events: _ -> [_ _]
      timeout: w1179 -> [_ _]
      tunnel: w1178 -> [_ w1190]
      event Timeout {
        n421 = event-data() -> ()  [unwired: 1 in, 3 out]
      }
      event "Jog Z": Value Change {
        n422 = event-data() -> ()  [unwired: 1 in, 1 out]
        n423 = property on="Steps /um" class="DigNum (strict)"() -> ("Value"=w1189:dbl)  [unwired: 2 in, 2 out]
        n424 = Multiply(x=w1189, y=10.0) -> (x*y=w1192:dbl)
        n425 = Format Into String(format string="movrel\\sz=%f\\s\\r\\n", w1192) -> (resulting string=w1193:string)  [unwired: 2 in, 1 out]
        n426 = VISA Write(VISA resource name=w1190, write buffer=w1193) -> ()  [unwired: 1 in, 3 out]
      }
    }
    n427 = event shown="[0] Timeout" {
      selector: _ -> [_ _]
      dyn-events: _ -> [_ _]
      timeout: w1179 -> [_ _]
      tunnel: w1185 -> [_ w1241]
      event Timeout {
        n428 = event-data() -> ()  [unwired: 1 in, 3 out]
      }
      event "405": Value Change {
        n429 = event-data() -> ("NewVal"=w1242:bool)  [unwired: 1 in, 5 out]
        n430 = call-poly <vilib>:"DAQmx Write.vi"("task/channels in"=w1241, "data"=w1242) -> ()  [unwired: 11 in, 3 out]
      }
    }
    n431 = event shown="[2] \"488 power\": Mouse Up" {
      selector: _ -> [_ _ _]
      dyn-events: _ -> [_ _ _]
      timeout: w1179 -> [_ _ _]
      tunnel: w1187 -> [_ w1219 _]
      tunnel: w1180 -> [_ _ w1224]
      event Timeout {
        n432 = event-data() -> ()  [unwired: 1 in, 3 out]
      }
      event "488": Value Change {
        n433 = event-data() -> ("NewVal"=w1220:bool)  [unwired: 1 in, 5 out]
        n434 = call-poly <vilib>:"DAQmx Write.vi"("task/channels in"=w1219, "data"=w1220) -> ()  [unwired: 11 in, 3 out]
      }
      event "488 power": Mouse Up {
        n435 = event-data() -> ()  [unwired: 1 in, 1 out]
        n436 = Divide(x="488 power", y=200.0) -> (x/y=w1221:dbl)
        n437 = stacked-sequence {
          seq-local: [w1225 _ _ _] -> [_ _ w1237 _]
          seq-local: [_ _ w1236 _] -> [_ _ _ w1239]
          tunnel: w1221 -> [w1226 _ _ _]
          tunnel: w1224 -> [_ w1231 _ w1240]
          frame #0 {
            w1230 = "p"  # Command
            n438 = Number To Fractional String(use system decimal point (T)=FALSE, number=w1226) -> (F-format string=w1228:string)  [unwired: 2 in]
            n439 = call <vilib>:"Space Constant.vi"() -> ("String"=w1229:string)
            n440 = Concatenate Strings(w1230, w1229, w1228) -> (w1225:string)
          }
          frame #1 {
            n441 = VISA Flush I/O Buffer(VISA resource name=w1231, mask (16)=u16 128) -> (VISA resource name out=w1234:refnum<visa-resource-name>, error out=w1235:errorcluster)  [unwired: 1 in]
            n442 = VISA Flush I/O Buffer(VISA resource name=w1234, mask (16)=u16 64, error in (no error)=w1235) -> ()  [unwired: 2 out]
          }
          frame #2 {
            w1238 = "\r"  # StopChar
            n443 = Concatenate Strings(w1237, w1238) -> (w1236:string)
          }
          frame #3 {
            n444 = VISA Write(VISA resource name=w1240, write buffer=w1239) -> ()  [unwired: 1 in, 3 out]
          }
        }
      }
    }
    n445 = event shown="[1] \"561\": Value Change" {
      selector: _ -> [_ _]
      dyn-events: _ -> [_ _]
      timeout: w1179 -> [_ _]
      tunnel: w1188 -> [_ w1217]
      event Timeout {
        n446 = event-data() -> ()  [unwired: 1 in, 3 out]
      }
      event "561": Value Change {
        n447 = event-data() -> ("NewVal"=w1218:bool)  [unwired: 1 in, 5 out]
        n448 = call-poly <vilib>:"DAQmx Write.vi"("task/channels in"=w1217, "data"=w1218) -> ()  [unwired: 11 in, 3 out]
      }
    }
    n449 = event shown="[1] \"647\": Value Change" {
      selector: _ -> [_ _ _]
      dyn-events: _ -> [_ _ _]
      timeout: w1179 -> [_ _ _]
      tunnel: w1182 -> [w1195 w1198 w1212]
      tunnel: [_ w1197 w1209] -> w1183
      tunnel: [w1195 w1196 w1210] -> w1184
      event Timeout {
        n450 = event-data() -> ()  [unwired: 1 in, 3 out]
      }
      event "647": Value Change {
        n451 = event-data() -> ("NewVal"=w1199:bool)  [unwired: 1 in, 5 out]
        n452 = case shown="True" w1199 {
          tunnel: w1198 -> [w1201 w1206]
          tunnel: [w1202 w1205] -> w1197
          tunnel: [w1200 w1204] -> w1196
          frame False {
            n453 = VISA Write(VISA resource name=w1201, write buffer="la off\r" ("format string")) -> (VISA resource name out=w1200:refnum<visa-resource-name>, error out=w1202:errorcluster)  [unwired: 1 in, 1 out]
          }
          frame True {
            n454 = VISA Write(VISA resource name=w1206, write buffer="la on\r" ("format string")) -> (VISA resource name out=w1204:refnum<visa-resource-name>, error out=w1205:errorcluster)  [unwired: 1 in, 1 out]
          }
        }
      }
      event "647 Power": Mouse Up {
        n455 = event-data() -> ()  [unwired: 1 in, 1 out]
        n456 = To Unsigned Byte Integer(number="647 Power") -> (unsigned 8bit integer=w1216:u8)
        n457 = Number To Decimal String(number=w1216) -> (decimal integer string=w1214:string)  [unwired: 1 in]
        n458 = Concatenate Strings("ch 1 pow ", w1214, "\r") -> (w1211:string)
        n459 = VISA Write(VISA resource name=w1212, write buffer=w1211) -> (VISA resource name out=w1210:refnum<visa-resource-name>, error out=w1209:errorcluster)  [unwired: 1 in, 1 out]
      }
    }
    n460 = property on="stop" class="Bool (strict)"() -> ("Value"=w1186:bool)  [unwired: 2 in, 2 out]
  }
  n461 = property class="MG17Motor"(reference="MG17Motor", "HWSerialNum"=i64 83839541 ("Numeric 2")) -> (reference out=w41:refnum<k7>)  [unwired: 1 in, 1 out]
  n462 = invoke class="MG17Motor" method="StartCtrl"(reference=w41) -> (reference out=w40:refnum<k7>, error out=w39:errorcluster)  [unwired: 2 in, 1 out]
  n463 = while {
    tunnel: w9 -> [w1253]
    tunnel: w10 -> [w1252]
    tunnel: w4 -> [w1254]
    tunnel: ["stop"] -> _
    tunnel: [w1254] -> w73
    tunnel: [w1253] -> w72
    tunnel: [w1252] -> w74
    shift-right: [w1246] -> _
    shift-left: 0 -> [w1245]
    tunnel: w17 -> [w1243]
    tunnel: [w1243] -> w16
    stop <- "stop" stop-if-true
    n464 = Greater?(x=w1245, y=8) -> (0:w1248:bool)
    n465 = Select(t=0, s=w1248, f=w1245) -> (s? t:f=w1247:i32)
    n466 = Add(x=1, y=w1247) -> (x+y=w1246:i32)
    "x+y" <- w1246
    n467 = case shown="True" "Go live" {
      tunnel: w1254 -> [_ w1261]
      tunnel: w1253 -> [_ w1260]
      tunnel: w1252 -> [_ w1259]
      tunnel: w1246 -> [_ w1256]
      frame False {
      }
      frame True {
        n468 = property on="561 voltages" class="Arr (strict)"() -> ("Value"=w1257:dbl[][])  [unwired: 2 in, 2 out]
        n469 = case shown="\"Static\", Default" "Live mode" {
          tunnel: w1257 -> [_ w1312 w1362 w1400]
          tunnel: w1260 -> [_ w1309 w1348 w1394]
          tunnel: w1259 -> [w1263 w1295 w1350 _]
          tunnel: w1261 -> [w1262 w1296 w1349 _]
          tunnel: w1256 -> [_ _ w1338 _]
          frame "Static", Default {
            n470 = flat-sequence {
              tunnel: w1263 -> [w1276]
              tunnel: [w1274] -> w1271
              tunnel: [w1273] -> w1270
              tunnel: w1262 -> [w1272]
              tunnel: [w1272] -> w1269
              tunnel: w1271 -> [w1280]
              tunnel: [w1280] -> w1268
              tunnel: w1270 -> [w1278]
              tunnel: [w1279] -> w1267
              tunnel: w1269 -> [w1279]
              tunnel: [w1278] -> w1266
              tunnel: w1268 -> [w1285]
              tunnel: [w1283] -> w1265
              tunnel: w1267 -> [w1283]
              tunnel: w1266 -> [w1282]
              tunnel: [w1281] -> w1264
              tunnel: w1265 -> [w1288]
              tunnel: w1264 -> [w1287]
              tunnel: [w1286] -> _
              frame #0 {
                n471 = call-poly <vilib>:"DAQmx Write.vi"("task/channels in"=w1276, "data"=TRUE) -> ("task out"=w1274:refnum<k21>, "error out"=w1273:errorcluster)  [unwired: 11 in, 1 out]
              }
              frame #1 {
                n472 = property on="Exposure time" class="DigNum (strict)"() -> ("Value"=w1277:dbl)  [unwired: 2 in, 2 out]
                n473 = Wait (ms)(milliseconds to wait=w1277) -> ()  [unwired: 1 out]
              }
              frame #2 {
                n474 = call-poly <vilib>:"DAQmx Write.vi"("task/channels in"=w1285, "data"=FALSE, "error in"=w1282) -> ("error out"=w1281:errorcluster)  [unwired: 10 in, 2 out]
              }
              frame #3 {
                n475 = while {
                  tunnel: w1288 -> [w1293]
                  tunnel: w1287 -> [w1292]
                  tunnel: [w1291] -> w1286
                  stop <- w1290 stop-if-true
                  n476 = call-poly <vilib>:"DAQmx Read.vi"("task/channels in"=w1293, "error in"=w1292) -> ("data"=w1289:bool, "error out"=w1291:errorcluster)  [unwired: 11 in, 1 out]
                  n477 = Not(x=w1289) -> (.not. x?=w1290:bool)
                }
              }
            }
          }
          frame "Widefield" {
            n478 = Index Array(array=w1312, index (row)=2, index (col)=1) -> ()  [unwired: 1 out]
            n479 = call <vilib>:"Triangle Waveform.vi"("offset"=1.0, "phase"=0.0, "amplitude"=0.06, "frequency"=0.1) -> ("signal out"=w1305:waveform(dbl))  [unwired: 6 in, 1 out]
            n480 = call-poly <vilib>:"DAQmx Write.vi"("task/channels in"=w1309, "data"=w1305) -> ()  [unwired: 11 in, 3 out]
            n481 = flat-sequence {
              tunnel: w1295 -> [w1317]
              tunnel: [w1315] -> w1304
              tunnel: [w1314] -> w1303
              tunnel: [w1313] -> w1302
              tunnel: w1296 -> [w1313]
              tunnel: w1304 -> [w1321]
              tunnel: [w1321] -> w1301
              tunnel: w1303 -> [w1319]
              tunnel: [w1320] -> w1300
              tunnel: w1302 -> [w1320]
              tunnel: [w1319] -> w1299
              tunnel: w1301 -> [w1326]
              tunnel: [w1324] -> w1298
              tunnel: w1300 -> [w1324]
              tunnel: w1299 -> [w1323]
              tunnel: [w1322] -> w1297
              tunnel: w1298 -> [w1329]
              tunnel: w1297 -> [w1328]
              tunnel: [w1327] -> _
              frame #0 {
                n482 = call-poly <vilib>:"DAQmx Write.vi"("task/channels in"=w1317, "data"=TRUE) -> ("task out"=w1315:refnum<k21>, "error out"=w1314:errorcluster)  [unwired: 11 in, 1 out]
              }
              frame #1 {
                n483 = property on="Exposure time" class="DigNum (strict)"() -> ("Value"=w1318:dbl)  [unwired: 2 in, 2 out]
                n484 = Wait (ms)(milliseconds to wait=w1318) -> ()  [unwired: 1 out]
              }
              frame #2 {
                n485 = call-poly <vilib>:"DAQmx Write.vi"("task/channels in"=w1326, "data"=FALSE, "error in"=w1323) -> ("error out"=w1322:errorcluster)  [unwired: 10 in, 2 out]
              }
              frame #3 {
                n486 = while {
                  tunnel: w1329 -> [w1334]
                  tunnel: w1328 -> [w1333]
                  tunnel: [w1332] -> w1327
                  stop <- w1331 stop-if-true
                  n487 = call-poly <vilib>:"DAQmx Read.vi"("task/channels in"=w1334, "error in"=w1333) -> ("data"=w1330:bool, "error out"=w1332:errorcluster)  [unwired: 11 in, 1 out]
                  n488 = Not(x=w1330) -> (.not. x?=w1331:bool)
                }
              }
            }
          }
          frame "SIM" {
            n489 = Quotient & Remainder(x=w1338, y=9) -> (x-y*floor(x/y)=w1360:i32)  [unwired: 1 out]
            n490 = flat-sequence {
              tunnel: w1349 -> [w1366]
              tunnel: w1350 -> [w1367]
              tunnel: [w1367] -> w1347
              tunnel: [w1363] -> w1345
              tunnel: [w1366] -> w1343
              tunnel: w1348 -> [w1365]
              tunnel: w1337 -> [w1364]
              tunnel: w1347 -> [w1371]
              tunnel: [w1371] -> w1346
              tunnel: w1345 -> [w1370]
              tunnel: [w1370] -> w1344
              tunnel: w1343 -> [w1369]
              tunnel: [w1369] -> w1342
              tunnel: [w1375] -> w1358
              tunnel: [w1373] -> w1357
              tunnel: [w1372] -> w1356
              tunnel: w1346 -> [w1377]
              tunnel: w1344 -> [w1374]
              tunnel: w1342 -> [w1372]
              tunnel: w1358 -> [w1381]
              tunnel: [w1381] -> w1355
              tunnel: w1357 -> [w1379]
              tunnel: [w1380] -> w1354
              tunnel: w1356 -> [w1380]
              tunnel: [w1379] -> w1353
              tunnel: w1355 -> [w1386]
              tunnel: [w1384] -> w1352
              tunnel: w1354 -> [w1384]
              tunnel: w1353 -> [w1383]
              tunnel: [w1382] -> w1351
              tunnel: w1352 -> [w1388]
              tunnel: w1351 -> [w1387]
              frame #0 {
                n491 = call-poly <vilib>:"DAQmx Write.vi"("task/channels in"=w1365, "data"=w1364) -> ("error out"=w1363:errorcluster)  [unwired: 11 in, 2 out]
              }
              frame #1 {
                n492 = property on="Settle time" class="DigNum (strict)"() -> ("Value"=w1368:u32)  [unwired: 2 in, 2 out]
                n493 = Wait (ms)(milliseconds to wait=w1368) -> ()  [unwired: 1 out]
              }
              frame #2 {
                n494 = call-poly <vilib>:"DAQmx Write.vi"("task/channels in"=w1377, "data"=TRUE, "error in"=w1374) -> ("task out"=w1375:refnum<k21>, "error out"=w1373:errorcluster)  [unwired: 10 in, 1 out]
              }
              frame #3 {
                n495 = property on="Exposure time" class="DigNum (strict)"() -> ("Value"=w1378:dbl)  [unwired: 2 in, 2 out]
                n496 = Wait (ms)(milliseconds to wait=w1378) -> ()  [unwired: 1 out]
              }
              frame #4 {
                n497 = call-poly <vilib>:"DAQmx Write.vi"("task/channels in"=w1386, "data"=FALSE, "error in"=w1383) -> ("error out"=w1382:errorcluster)  [unwired: 10 in, 2 out]
              }
              frame #5 {
                n498 = while {
                  tunnel: w1388 -> [w1393]
                  tunnel: w1387 -> [w1392]
                  tunnel: [w1391] -> _
                  stop <- w1390 stop-if-true
                  n499 = call-poly <vilib>:"DAQmx Read.vi"("task/channels in"=w1393, "error in"=w1392) -> ("data"=w1389:bool, "error out"=w1391:errorcluster)  [unwired: 11 in, 1 out]
                  n500 = Not(x=w1389) -> (.not. x?=w1390:bool)
                }
              }
            }
            n501 = Add(x=0, y=w1360) -> (x+y=w1339:i32)
            n502 = Index Array(array=i32[] [1, 2, 0, 1, 2, 0, 1, 2, 0, 0, 1, 2, 3, 4, 0], index=w1339) -> (element=w1335:i32)
            n503 = Index Array(array=i32[] [0, 0, 1, 1, 1, 2, 2, 2, 0, 2, 2, 2, 2, 2, 0], index=w1339) -> (element=w1336:i32)
            n504 = Index Array(array=w1362, index (row)=w1335, index (col)=w1336) -> (element=w1337:dbl)
            n505 = property on="Current voltage" class="DigNum (strict)"("Value"=w1337) -> ()  [unwired: 2 in, 2 out]
          }
          frame "Strobe" {
            n506 = flat-sequence {
              tunnel: w1400 -> [w1402]
              tunnel: [w1402] -> w1398
              tunnel: w1394 -> [w1401]
              tunnel: [w1407] -> w1399
              tunnel: w1398 -> [w1407]
              tunnel: w1399 -> [w1409]
              tunnel: [w1409] -> w1397
              tunnel: w1394 -> [w1408]
              tunnel: w1397 -> [w1414]
              tunnel: [w1414] -> w1396
              tunnel: w1396 -> [w1416]
              tunnel: [w1416] -> w1395
              tunnel: w1394 -> [w1415]
              tunnel: [w1421] -> _
              tunnel: w1395 -> [w1421]
              frame #0 {
                n507 = Index Array(array=w1402, index (row)=2, index (col)=0) -> (element=w1403:dbl)
                n508 = call-poly <vilib>:"DAQmx Write.vi"("task/channels in"=w1401, "data"=w1403) -> ()  [unwired: 11 in, 3 out]
              }
              frame #1 {
                n509 = property on="Settle time" class="DigNum (strict)"() -> ("Value"=w1406:u32)  [unwired: 2 in, 2 out]
                n510 = Wait (ms)(milliseconds to wait=w1406) -> ()  [unwired: 1 out]
              }
              frame #2 {
                n511 = Index Array(array=w1409, index (row)=2, index (col)=1) -> (element=w1412:dbl)
                n512 = call-poly <vilib>:"DAQmx Write.vi"("task/channels in"=w1408, "data"=w1412) -> ()  [unwired: 11 in, 3 out]
              }
              frame #3 {
                n513 = property on="Settle time" class="DigNum (strict)"() -> ("Value"=w1413:u32)  [unwired: 2 in, 2 out]
                n514 = Wait (ms)(milliseconds to wait=w1413) -> ()  [unwired: 1 out]
              }
              frame #4 {
                n515 = Index Array(array=w1416, index (row)=2, index (col)=2) -> (element=w1417:dbl)
                n516 = call-poly <vilib>:"DAQmx Write.vi"("task/channels in"=w1415, "data"=w1417) -> ()  [unwired: 11 in, 3 out]
              }
              frame #5 {
                n517 = property on="Settle time" class="DigNum (strict)"() -> ("Value"=w1420:u32)  [unwired: 2 in, 2 out]
                n518 = Wait (ms)(milliseconds to wait=w1420) -> ()  [unwired: 1 out]
              }
            }
          }
        }
      }
    }
    "?" <- "Go live"
  }
  n519 = stacked-sequence {
    tunnel: w40 -> [w1424 w1442]
    tunnel: w39 -> [w1423 _]
    tunnel: [_ w1441] -> w38
    tunnel: [_ w1440] -> _
    frame #0 {
      n520 = invoke class="MG17Motor" method="SetVelParams"(reference=w1424, error in=w1423, "lChanID"=0, "fMinVel"=0.0, "fAccn"=20, "fMaxVel"=20) -> (reference out=w1431:refnum<k7>, error out=w1430:errorcluster)  [unwired: 1 in, 5 out]
      n521 = property on="561 power" class="Slide (strict)"() -> ("Value"=w1426:dbl)  [unwired: 2 in, 2 out]
      n522 = Multiply(x=45, y=w1426) -> (x*y=w1427:dbl)
      n523 = Add(x=78, y=w1427) -> (x+y=w1425:dbl)
      n524 = invoke class="MG17Motor" method="SetAbsMovePos"(reference=w1431, error in=w1430, "lChanID"=0, "fAbsPos"=w1425) -> (reference out=w1433:refnum<k7>, error out=w1432:errorcluster)  [unwired: 1 in, 3 out]
      n525 = invoke class="MG17Motor" method="MoveAbsolute"(reference=w1433, error in=w1432, "lChanID"=0, "bWait"=TRUE) -> ()  [unwired: 1 in, 5 out]
    }
    frame #1 {
      n526 = while {
        tunnel: [w1451] -> w1441
        tunnel: w1442 -> [w1449]
        tunnel: [w1448] -> w1440
        stop <- w1447 stop-if-true
        n527 = Wait (ms)(milliseconds to wait=250) -> ()  [unwired: 1 out]
        n528 = Divide(x="561 power", y=100.0) -> (x/y=w1443:dbl)
        n529 = event shown="[0] Timeout" {
          selector: _ -> [_ _]
          dyn-events: _ -> [_ _]
          timeout: 10 -> [_ _]
          tunnel: w1449 -> [w1452 w1460]
          tunnel: [w1452 w1459] -> w1451
          tunnel: w1443 -> [_ w1455]
          tunnel: [_ w1462] -> w1448
          event Timeout {
            n530 = event-data() -> ()  [unwired: 1 in, 3 out]
          }
          event "561 power": Mouse Up {
            n531 = event-data() -> ()  [unwired: 1 in, 4 out]
            n532 = Multiply(x=45, y=w1455) -> (x*y=w1456:dbl)
            n533 = Add(x=81 ("561 power offset"), y=w1456) -> (x+y=w1454:dbl)
            n534 = invoke class="MG17Motor" method="SetAbsMovePos"(reference=w1460, "lChanID"=0, "fAbsPos"=w1454) -> (reference out=w1458:refnum<k7>)  [unwired: 2 in, 4 out]
            n535 = invoke class="MG17Motor" method="MoveAbsolute"(reference=w1458, "lChanID"=0, "bWait"=TRUE) -> (reference out=w1459:refnum<k7>, error out=w1462:errorcluster)  [unwired: 2 in, 3 out]
          }
        }
        n536 = property on="stop" class="Bool (strict)"() -> ("Value"=w1447:bool)  [unwired: 2 in, 2 out]
      }
    }
  }
  n537 = invoke class="MG17Motor" method="StopCtrl"(reference=w38) -> ()  [unwired: 2 in, 3 out]
  n538 = VISA Close(VISA resource name=w6) -> (error out=w5:errorcluster)  [unwired: 1 in]
  n539 = call <vilib>:"DAQmx Stop Task.vi"("task/channels in"=w16) -> ("task out"=w15:refnum<k21>)  [unwired: 13 in, 1 out]
  n540 = VISA Close(VISA resource name=w45, error in (no error)=w44) -> (error out=w43:errorcluster)
  n541 = call <vilib>:"DAQmx Clear Task.vi"("task in"=w15) -> ("error out"=w14:errorcluster)  [unwired: 14 in]
  n542 = call <vilib>:"DAQmx Stop Task.vi"("task/channels in"=w74) -> ("task out"=w69:refnum<k21>)  [unwired: 13 in, 1 out]
  n543 = call <vilib>:"DAQmx Stop Task.vi"("task/channels in"=w72) -> ("task out"=w71:refnum<k21>)  [unwired: 13 in, 1 out]
  n544 = call-poly <vilib>:"DAQmx Write.vi"("task/channels in"=w64, "data"=w63) -> ("task out"=w60:refnum<k21>, "error out"=w58:errorcluster)  [unwired: 11 in, 1 out]
  n545 = call-poly <vilib>:"DAQmx Write.vi"("task/channels in"=w65, "data"=w63) -> ("task out"=w59:refnum<k21>, "error out"=w57:errorcluster)  [unwired: 11 in, 1 out]
  n546 = call <vilib>:"DAQmx Stop Task.vi"("task/channels in"=w73) -> ("task out"=w70:refnum<k21>)  [unwired: 13 in, 1 out]
  n547 = call <vilib>:"DAQmx Clear Task.vi"("task in"=w69) -> ("error out"=w28:errorcluster)  [unwired: 14 in]
  n548 = call <vilib>:"DAQmx Clear Task.vi"("task in"=w71) -> ("error out"=w67:errorcluster)  [unwired: 14 in]
  n549 = property on="Go live" class="Bool (strict)"(error in=w28, "Value"=FALSE) -> (error out=w27:errorcluster)  [unwired: 1 in, 1 out]
  n550 = call <vilib>:"DAQmx Clear Task.vi"("task in"=w70) -> ("error out"=w66:errorcluster)  [unwired: 14 in]
  n551 = call <vilib>:"DAQmx Stop Task.vi"("task/channels in"=w60, "error in"=w58) -> ("task out"=w61:refnum<k21>, "error out"=w55:errorcluster)  [unwired: 12 in]
  n552 = call <vilib>:"DAQmx Stop Task.vi"("task/channels in"=w59, "error in"=w57) -> ("task out"=w62:refnum<k21>, "error out"=w56:errorcluster)  [unwired: 12 in]
  n553 = Merge Errors(w67, w66, w27, w14) -> (→"Camera/galvo error":errorcluster)
  n554 = call <vilib>:"DAQmx Clear Task.vi"("task in"=w62, "error in"=w56) -> ("error out"=w53:errorcluster)  [unwired: 13 in]
  n555 = call <vilib>:"DAQmx Clear Task.vi"("task in"=w61, "error in"=w55) -> ("error out"=w54:errorcluster)  [unwired: 13 in]
  n556 = Merge Errors(w53, w54, w43, w5) -> (→"Laser error":errorcluster)
  n557 = VISA Close(VISA resource name=w51) -> ()  [unwired: 1 in, 1 out]
